vi "MainGUI.vi"() -> ()   [LabVIEW 2018]
uses:
  General/Controls/ScanType.ctl
  General/Controls/Vibratome Parameters.ctl
  General/Controls/Imaging Parameters.ctl
  General/Controls/Scan Direction.ctl
  General/type defines/Alazar parameters.ctl
  Hardware Mfg/AlazarTech SDK/Controls/General Trigger Settings.ctl
  Hardware Mfg/AlazarTech SDK/Controls/Trigger Engine Controls.ctl
  Hardware Mfg/AlazarTech SDK/Controls/Alazar Device ID.ctl
  Hardware Mfg/AlazarTech SDK/Controls/Channel Input Controls.ctl
  Hardware Mfg/AlazarTech SDK/Controls/Alazar Acquisition Settings.ctl
  Hardware Mfg/AlazarTech SDK/Controls/Clock Controls.ctl
  General/Controls/Optical Parameters.ctl
  General/Controls/Translation Stage Parameters.ctl
  Hardware Mfg/Thorlabs Translation Stages/Controls/Translation Stage Cluster.ctl
  General/Controls/Translation Stage Types.ctl
  General/type defines/Manual Controls.ctl
  General/type defines/FFT parameters.ctl
  General/type defines/FFT mode.ctl
  General/type defines/Vibratome Param.ctl
  General/Controls/Queue Manager Actions.ctl
  General/Controls/MessagePacket.ctl
  General/Controls/QueueNames.ctl
  General/Controls/FGV Actions.ctl
  General/Controls/Save Bline to Mem Control.ctl
  General/Tile naming actions.ctl
  Hardware Mfg/Main Scan Processor Status.vi
  Hardware Mfg/Axsun Laser/Axsun action.ctl
panel:
  in  "Status":string
  in  "Quit":bool
  in  "Acquire":bool
  in  "Control Panel":T1(tab)
  in  "Optical Parameters":T2={"Obj. Focal Length [mm]"=45.0, "Scan Lens EFL[mm]"=59.5, "Tube Lens EFL[mm]"=205.0, "Galvo V Range (+/-)"=10.0, "Galvo Max Half Angle [Deg]"=19.0, "Max Galvo Range[%]"=0.0}
  in  "Galvo HW Parameters":T3={"Analog Out Channel"="GalvoCtrl/ao0,GalvoCtrl/ao1", "Min Voltage"=-10.0, "Max Voltage"=10.0, "Pixel Clock Source"="/GalvoCtrl/PFI0", "Sample Rate"=1000.0, "Line Clock Out Ch"="GalvoCtrl/port0/line0"}
  in  "Imaging Parameter":T4={"Raster Scan Direction"=enum."Uni Directional", "Pixel Dwell Time [Clock Cycles]"=1, "Flyback Time [Clock Cycles]"=150, "XY Center [um]"={"X"=550.0, "Y"=450.0}, "Pixel Step Size [um] X"=3.0, "XY Image Size"=enum."2048 x 2048", "Custom"=TRUE, "Custom Size"={"X"=1050, "Y"=30}, "Line Averages"=1, "Pixel Step Size [um] Y"=0.0} {"Pixel Step Size [um] Y" min=0.0 max=10.0 step=0.01; "Line Averages" min=1 max=30 step=1; "Flyback Time [Clock Cycles]" max=1000 step=1; "Pixel Step Size [um] X" min=0.0 max=100.0 step=0.01; "Custom Size"."Y" min=2 max=10000 step=1; "Custom Size"."X" min=1 max=30 step=1; "XY Center [um]"."Y" min=1.0 max=30.0 step=1.0; "XY Center [um]"."X" min=1.0 max=30.0 step=1.0; "Pixel Dwell Time [Clock Cycles]" max=10 step=1}
  in  "Scan Type":T6
  in  "Alazar parameters":T7={"Trigger Settings"={"General Trigger Settings"={"Trigger Operation"=0, "Coupling ID"=2, "Range ID"=2, "Delay"=0, "Timeout Ticks"=0, "Mode"=1, "Parameter"=1}, "Trigger Engine 1"={"Trigger Engine"=0, "Source"=2, "Slope"=1, "Level"=140}, "Trigger Engine 2"={"Trigger Engine"=1, "Source"=2, "Slope"=1, "Level"=2048}}, "Device ID"={"System ID"=1, "Board ID"=1}, "Ch A Input Control"={"Channel"=1, "Coupling"=2, "Range"=7, "Impedance"=2}, "Ch B Input Control"={"Channel"=2, "Coupling"=2, "Range"=7, "Impedance"=2}, "Acq Settings"={"Record Length"=1440, "Offset"=0, "Records Per Buffer"=1100, "Records Count (Records/Acq)"=2147483647, "Window Type"=1, "Footer"=0, "Samples per record"=2048, "Output Format"=11}, "Capture Clock"={"Sample Rate"=100, "Decimation"=0, "Source"=2, "Edge"=0}} {"Capture Clock"."Edge" items=["Rising", "Falling"]; "Capture Clock"."Source" items=["Internal"=1, "Fast External"=2, "Medium External"=3, "Slow External"=4, "External AC"=5, "External DC"=6, "External 10MHz"=7]; "Acq Settings"."Output Format" items=["Float Log"=11, "Float Amp"=10, "U16_LOG"=1, "U16_AMP2"=257, "Real"=3, "Imag"=4]; "Acq Settings"."Footer" items=["FOOTER_NONE", "FOOTER_NPT"]; "Acq Settings"."Window Type" items=["DSP_WINDOW_NONE", "DSP_WINDOW_HANNING", "DSP_WINDOW_HAMMING", "DSP_WINDOW_BLACKMAN", "DSP_WINDOW_BLACKMAN_HARRIS", "DSP_WINDOW_BARTLETT"]; "Ch B Input Control"."Channel" items=["A"=1, "B"=2, "C"=4, "D"=8]; "Ch B Input Control"."Coupling" items=["AC"=1, "DC"=2]; "Ch B Input Control"."Range" items=["20 mV"=1, "40 mV"=2, "50 mV"=3, "80 mV"=4, "100 mV"=5, "200 mV"=6, "400 mV"=7, "500 mV"=8, "800 mV"=9, "1 V"=10, "1.25 V"=33, "2 V"=11, "4 V"=12, "5 V"=13, "8 V"=14, "10 V"=15, "20 V"=16]; "Ch B Input Control"."Impedance" items=["1 MOhm"=1, "50 Ohm"=2, ""=0]; "Ch A Input Control"."Channel" items=["A"=1, "B"=2, "C"=4, "D"=8]; "Ch A Input Control"."Coupling" items=["AC"=1, "DC"=2]; "Ch A Input Control"."Range" items=["20 mV"=1, "40 mV"=2, "50 mV"=3, "80 mV"=4, "100 mV"=5, "200 mV"=6, "400 mV"=7, "500 mV"=8, "800 mV"=9, "1 V"=10, "1.25 V"=33, "2 V"=11, "4 V"=12, "5 V"=13, "8 V"=14, "10 V"=15, "20 V"=16]; "Ch A Input Control"."Impedance" items=["1 MOhm"=1, "50 Ohm"=2, ""=0]; "Trigger Settings"."General Trigger Settings"."Trigger Operation" items=["J", "K", "J OR K", "J AND K", "J XOR K", "J AND NOT K", "NOT J AND K"]; "Trigger Settings"."General Trigger Settings"."Coupling ID" items=["AC"=1, "DC"=2]; "Trigger Settings"."General Trigger Settings"."Range ID" items=["5 V", "1 V", "TTL"]; "Trigger Settings"."Trigger Engine 1"."Trigger Engine" items=["J", "K"]; "Trigger Settings"."Trigger Engine 1"."Source" items=["A", "B", "External", "Disable", "C", "D"]; "Trigger Settings"."Trigger Engine 1"."Slope" items=["Positive"=1, "Negative"=2]; "Trigger Settings"."Trigger Engine 2"."Trigger Engine" items=["J", "K"]; "Trigger Settings"."Trigger Engine 2"."Source" items=["A", "B", "External", "Disable", "C", "D"]; "Trigger Settings"."Trigger Engine 2"."Slope" items=["Positive"=1, "Negative"=2]}
  in  "Vibratome Axis":T14={"Start [mm](first cut height)"=45.85, "slice thickness[um]"=2.1, "#slice"=111, "slice thick2[um]"=2.1, "#thin slices"=111, "image thickness(um)"=0.0, "#images"=0, "image depth2"=0.0, "#image depth2"=0}
  in  "Vibratome":T15={"Z Bottom [mm]"=0.0, "Pre Cut Dwell [s]"=0.0, "Blade Frequency [RPM]"=0, "Slice Speed [mm/s]"=0.0, "Post Cut Dwell [s]"=0.0, "Ramp Time [s]"=0.0, "Start X [mm]"=0.0, "Start Y [mm]"=0.0, "Slice Length [mm]"=0.0, "Slice Axis"=enum."X Axis", "Controller VISA Ref"="COM4"}
  in  "Mosaic Paramter":T16={"X Axis"={"Start [mm]"=56.0, "FOV[mm]"=3.0, "End [mm]"=70.8}, "Y Axis"={"Start [mm]"=102.5, "FOV[mm]"=3.0, "End [mm]"=117.2}, "Scan Pattern"=enum."Uni-directional", "Overlap Options"={"Overlap Type"=enum."X and Y", "Percent Overlap"=10, "Justify"=enum."Start"}}
  out "Current Position out":cluster{"X":dbl, "Y":dbl}
  in  "Manual Controls":T17={"Z0"=10.0, "First image height"=0.0, "Data Path"=path "C:/Users/BOAS-USER/Documents/Data/0922", "Save parameters"={"start pixel"=45, "#pixels to save"=100}, "Center Galvos"=FALSE, "Acquisition mode"=enum."Alazar FFT", "PSOCT Channel"=1, "Save"=FALSE, "AIP rotation angle"=0.0, "Scan Parameters"={"# Scan"={"#Ascan"=150, "#Bscan"=400}, "# Rpt"={"#ARpt"=1, "#BRpt"=1}, "Aline Rate"=2, "# Extra"={"# ARpt_extra"=5, "#Brtn_extra"=60}}, "ROI Parameters"={"ROI (mm)"={"X (mm)"=1.0, "Y (mm)"=1.0}, "Shift (mm)"={"Xshift (mm)"=0.0, "Yshift (mm)"=0.0}}, "Objective"=30} {"Objective" items=["5X LKM05", "10X LKM10", "20X LKM20", "10X LSM02"]; "Scan Parameters"."Aline Rate" items=["76 KHz", "146 KHz", "76 KHz", "28 KHz", "10 KHz"]; "PSOCT Channel" items=["A"=1, "B"=2, "A + B"=3, "C"=4, "A + C"=5, "A + B"=6, "D"=8, "A + D"=9, "B + D"=10, "C + D"=12, "A + B + C + D"=15]}
  out "image plane out":dbl
  out "slice plane out":dbl
  in  "Table Stages":T20={"X Stage"={"Position"=0.0, "Is.Enabled?"=FALSE, "Is.Connected?"=FALSE, "Device SN"="45876425", "AccelerationMaximum"=20.0, "VelocityMaximum"=20.0, "Acceleration"=10.0, "Velocity"=10.0, "waitTimeout (ms)"=1000000, "Model"=enum."Thorlabs LTS", "Is.Homed?"=FALSE}, "Y Stage"={"Position"=0.0, "Is.Enabled?"=FALSE, "Is.Connected?"=FALSE, "Device SN"="45995820", "AccelerationMaximum"=20.0, "VelocityMaximum"=20.0, "Acceleration"=10.0, "Velocity"=10.0, "waitTimeout (ms)"=10000000, "Model"=enum."Thorlabs LTS", "Is.Homed?"=FALSE}, "Z Stage"={"Position"=0.0, "Is.Enabled?"=FALSE, "Is.Connected?"=FALSE, "Device SN"="49103464", "AccelerationMaximum"=8.0, "VelocityMaximum"=3.0, "Acceleration"=4.0, "Velocity"=2.0, "waitTimeout (ms)"=1000000, "Model"=enum."Thorlabs MLJ", "Is.Homed?"=FALSE}}
  out "XY Graph out":cluster{"X":dbl, "Y":dbl}[](graph)
  out "AIP":T23(plugin-control) caption="Image"
  # "Image Settings"
  # "Optical Settings"
  # "X"
  # "X"
  # "Vibratome Settings"
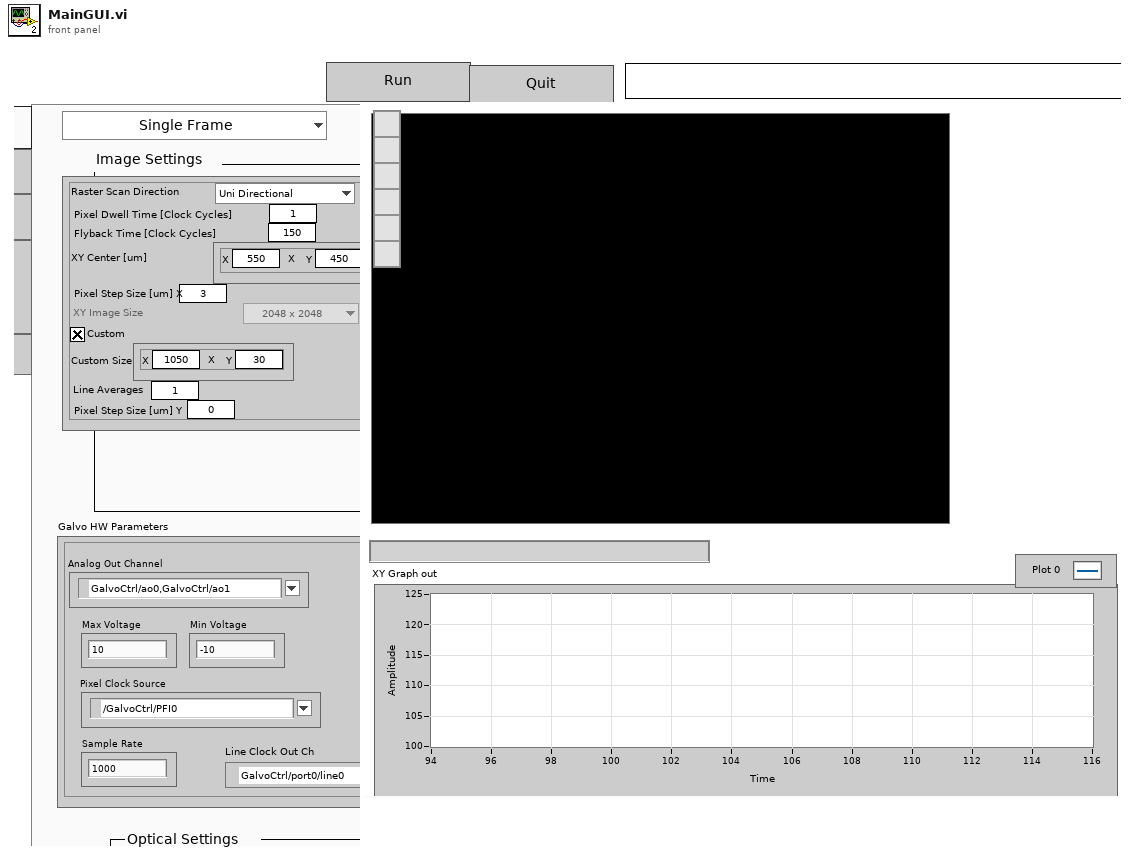
[diagram p1: front panel]
types:
  T1 = enum32{"Galvo", "Alazar", "Config", "Manual Contorls", "Table"}
  T2 = typedef "Optical Parameters.ctl" = cluster{"Obj. Focal Length [mm]":dbl, "Scan Lens EFL[mm]":dbl, "Tube Lens EFL[mm]":dbl, "Galvo V Range (+/-)":dbl, "Galvo Max Half Angle [Deg]":dbl, "Max Galvo Range[%]":dbl}
  T3 = cluster{"Analog Out Channel":tag, "Min Voltage":dbl, "Max Voltage":dbl, "Pixel Clock Source":tag, "Sample Rate":dbl, "Line Clock Out Ch":tag}
  T4 = typedef "Imaging Parameters.ctl" = cluster{"Raster Scan Direction":T5, "Pixel Dwell Time [Clock Cycles]":u16, "Flyback Time [Clock Cycles]":u16, "XY Center [um]":cluster{"X":dbl, "Y":dbl}, "Pixel Step Size [um] X":dbl, "XY Image Size":enum16{"32 x 32", "64 x 64", "128 x 128", "256 x 256", "512 x 512", "1024 x 1024", "2048 x 2048"}, "Custom":bool, "Custom Size":cluster{"X":u16, "Y":u16}, "Line Averages":u8, "Pixel Step Size [um] Y":dbl}
  T5 = typedef "Scan Direction.ctl" = enum16{"Uni Directional", "Bi Directional", "None"}
  T6 = typedef "ScanType.ctl" = enum16{"Single Frame", "Continuous Frame", "ROI Line", "Vibratome", "Mosaic", "Mosaic + Slice"}
  T7 = typedef "Alazar parameters.ctl" = cluster{"Trigger Settings":cluster{"General Trigger Settings":T8, "Trigger Engine 1":T9, "Trigger Engine 2":T9}, "Device ID":T10, "Ch A Input Control":T11, "Ch B Input Control":T11, "Acq Settings":T12, "Capture Clock":T13}
  T8 = typedef "General Trigger Settings.ctl" = cluster{"Trigger Operation":u32, "Coupling ID":u32, "Range ID":u32, "Delay":u32, "Timeout Ticks":u32, "Mode":u32, "Parameter":u32}
  T9 = typedef "Trigger Engine Controls.ctl" = cluster{"Trigger Engine":u32, "Source":u32, "Slope":u32, "Level":u32}
  T10 = typedef "Alazar Device ID.ctl" = cluster{"System ID":u32, "Board ID":u32}
  T11 = typedef "Channel Input Controls.ctl" = cluster{"Channel":u8, "Coupling":u32, "Range":u32, "Impedance":u32}
  T12 = typedef "Alazar Acquisition Settings.ctl" = cluster{"Record Length":u32, "Offset":u32, "Records Per Buffer":u32, "Records Count (Records/Acq)":u32, "Window Type":u32, "Footer":u32, "Samples per record":u32, "Output Format":u32}
  T13 = typedef "Clock Controls.ctl" = cluster{"Sample Rate":u32, "Decimation":u32, "Source":u32, "Edge":u32}
  T14 = typedef "Vibratome Param.ctl" = cluster{"Start [mm](first cut height)":dbl, "slice thickness[um]":dbl, "#slice":u16, "slice thick2[um]":dbl, "#thin slices":u16, "image thickness(um)":dbl, "#images":u16, "image depth2":dbl, "#image depth2":u16}
  T15 = typedef "Vibratome Parameters.ctl" = cluster{"Z Bottom [mm]":dbl, "Pre Cut Dwell [s]":dbl, "Blade Frequency [RPM]":u16, "Slice Speed [mm/s]":dbl, "Post Cut Dwell [s]":dbl, "Ramp Time [s]":dbl, "Start X [mm]":dbl, "Start Y [mm]":dbl, "Slice Length [mm]":dbl, "Slice Axis":enum16{"X Axis", "Y Axis", "Z Axis"}, "Controller VISA Ref":refnum<visa-resource-name>}
  T16 = cluster{"X Axis":cluster{"Start [mm]":dbl, "FOV[mm]":dbl, "End [mm]":dbl}, "Y Axis":cluster{"Start [mm]":dbl, "FOV[mm]":dbl, "End [mm]":dbl}, "Scan Pattern":enum16{"Uni-directional", "Bi-Directional", "Spiral Out", "Spiral In"}, "Overlap Options":cluster{"Overlap Type":enum16{"No Overlap", "X Only", "Y Only", "X and Y"}, "Percent Overlap":u8, "Justify":enum16{"Start", "Center", "End"}}}
  T17 = typedef "Manual Controls.ctl" = cluster{"Z0":dbl, "First image height":dbl, "Data Path":path, "Save parameters":T18, "Center Galvos":bool, "Acquisition mode":T19, "PSOCT Channel":u32, "Save":bool, "AIP rotation angle":dbl, "Scan Parameters":cluster{"# Scan":cluster{"#Ascan":i32, "#Bscan":i32}, "# Rpt":cluster{"#ARpt":i32, "#BRpt":i32}, "Aline Rate":u16, "# Extra":cluster{"# ARpt_extra":i32, "#Brtn_extra":i32}}, "ROI Parameters":cluster{"ROI (mm)":cluster{"X (mm)":dbl, "Y (mm)":dbl}, "Shift (mm)":cluster{"Xshift (mm)":sgl, "Yshift (mm)":sgl}}, "Objective":u16}
  T18 = typedef "FFT parameters.ctl" = cluster{"start pixel":i32, "#pixels to save":i32}
  T19 = typedef "FFT mode.ctl" = enum16{"ThorOCT B line", "ThorOCT Spectral", "ThorOCT FFT", "Alazar B line", "Alazar FFT", "GPU FFT", "Alazar Spectral"}
  T20 = typedef "Translation Stage Parameters.ctl" = cluster{"X Stage":T21, "Y Stage":T21, "Z Stage":T21}
  T21 = typedef "Translation Stage Cluster.ctl" = cluster{"Position":dbl, "Is.Enabled?":bool, "Is.Connected?":bool, "Device SN":string, "AccelerationMaximum":dbl, "VelocityMaximum":dbl, "Acceleration":dbl, "Velocity":dbl, "waitTimeout (ms)":i32, "Model":T22, "Is.Homed?":bool}
  T22 = typedef "Translation Stage Types.ctl" = enum16{"None", "Thorlabs LTS", "Thorlabs MLJ"}
  T23 = typedef "IMAQ Image.ctl" = refnum<image>
  T24 = typedef "Queue Manager Actions.ctl" = enum16{"Init", "Enqueue", "Enqueue All", "Preview Queue", "Dequeue", "Get Status", "Flush Queue", "Flush All Queues", "Release All Queues", "Release Queue", "Enqueue at Opposite End"}
  T25 = typedef "QueueNames.ctl" = enum16{"Main GUI", "Main Scan Processor", "Main Processing", "Main Saving", "Main Display", "Main Table Stage GUI", "Main Table Stage Proc.", "Scan Engine", "Vibratome GUI", "Vibratome Processor", "Slice Engine"}
  T26 = typedef "MessagePacket.ctl" = cluster{"Message":string, "Parameter":variant}
  T27 = typedef "FGV Actions.ctl" = enum16{"Init", "Set", "Get", "Clear"}
  T28 = typedef "Image Type" = u32
  T29 = typedef "System Parameters.ctl" = cluster{"Optical Parameters":T2, "Vibratome":T15, "Table Stages":T20, "Imaging Parameter":T4, "Galvo HW Parameters":cluster{"Analog Out Channel":tag, "Min Voltage":dbl, "Max Voltage":dbl, "Pixel Clock Source":tag, "Sample Rate":dbl, "Line Clock Out Ch":tag}, "Alazar parameters":T7, "Mosaic Paramter":cluster{"X Axis":cluster{"Start [mm]":dbl, "Steps [pts]":dbl, "End [mm]":dbl}, "Y Axis":cluster{"Start [mm]":dbl, "Steps [pts]":dbl, "End [mm]":dbl}, "Scan Pattern":enum16{"Uni-directional", "Bi-Directional", "Spiral Out", "Spiral In"}, "Overlap Options":cluster{"Overlap Type":enum16{"No Overlap", "X Only", "Y Only", "X and Y"}, "Percent Overlap":u8, "Justify":enum16{"Start", "Center", "End"}}}, "Manual Controls":T17, "Vibratome Axis":T14}
  T30 = typedef "Tile naming actions.ctl" = enum16{"Export", "Increment", "Total tile num", "Init"}
  T31 = typedef "Axsun action.ctl" = enum16{"GetSystemStatus", "Clock delay", "GetLaserOnTime", "GetWaveLengthAtSweptTrigger", "Source current ON", "GetSerialNum", "GetControlVersion", "Laser ON", "Laser OFF", "Source current OFF", "Get laser handle", "Start Network Control Interface", "stop", "Create handle"}
  T32 = typedef "Save Bline to Mem Control.ctl" = enum16{"Output data", "Save(ThorOCT)", "Save(PSOCT)", "FFT and Save", "Uninit", "PSOCT Spectral buffer Set", "PSOCT Spatial buffer Set", "PSOCT Spectral buffer Init", "PSOCT Spatial buffer Init", "ThorOCT Spectral buffer Init", "ThorOCT Spatial buffer Init", "ThorOCT Spectral buffer Set", "ThorOCT Spatial buffer Set", "ThorOCT Spectral Save", "Alazar Spectral Save"}
  T33 = cluster{"X Axis":cluster{"Start [mm]":dbl, "Steps [pts]":dbl, "End [mm]":dbl}, "Y Axis":cluster{"Start [mm]":dbl, "Steps [pts]":dbl, "End [mm]":dbl}, "Scan Pattern":enum16{"Uni-directional", "Bi-Directional", "Spiral Out", "Spiral In"}, "Overlap Options":cluster{"Overlap Type":enum16{"No Overlap", "X Only", "Y Only", "X and Y"}, "Percent Overlap":u8, "Justify":enum16{"Start", "Center", "End"}}}
  T34 = enum16{"32 x 32", "64 x 64", "128 x 128", "256 x 256", "512 x 512", "1024 x 1024", "2048 x 2048"}
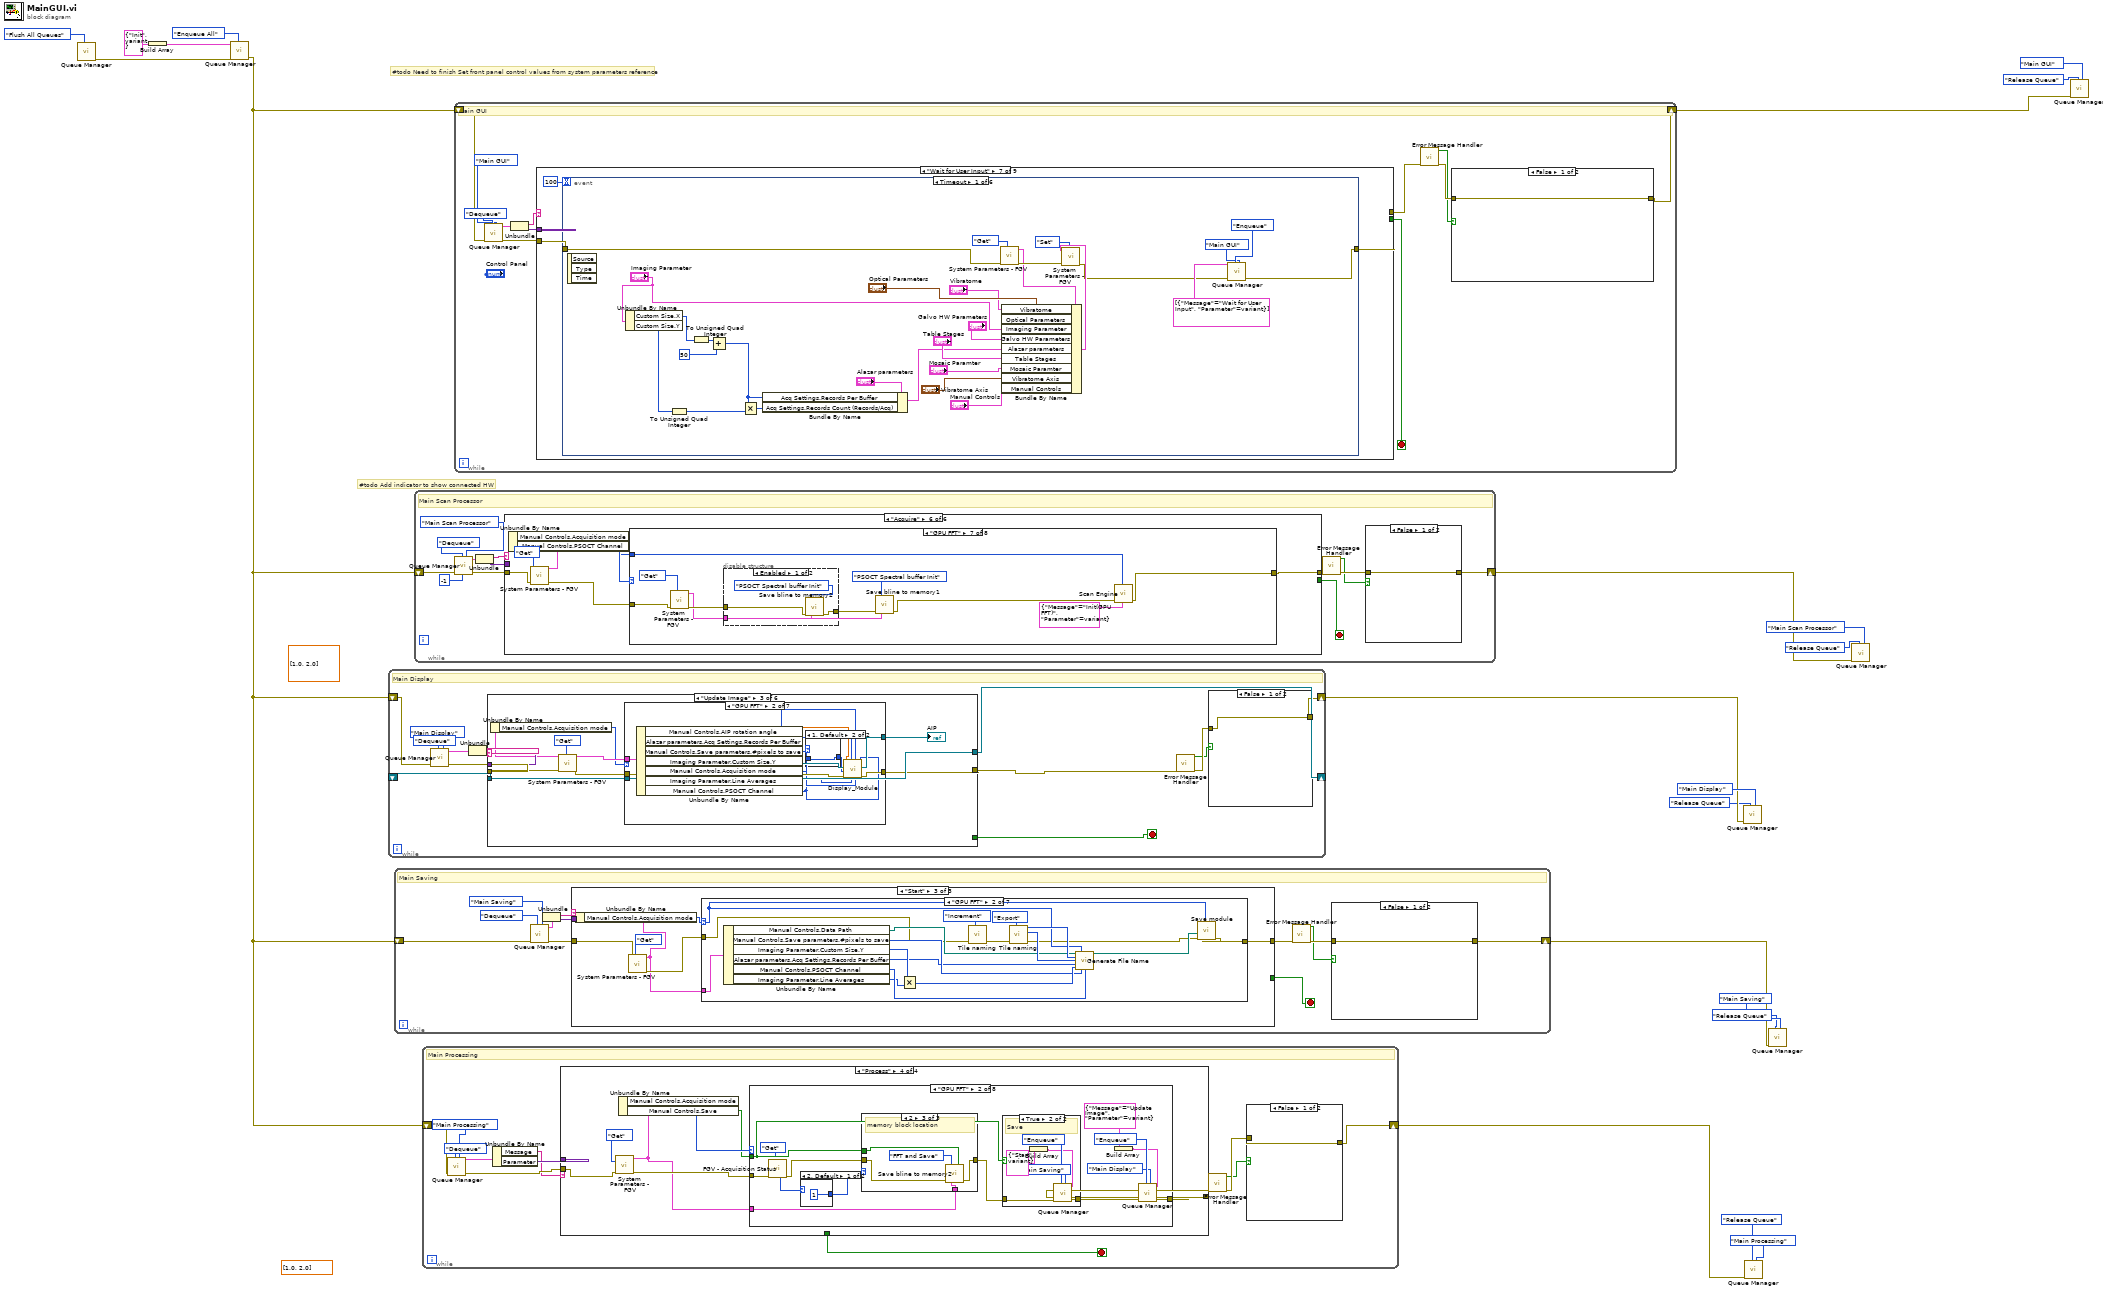
[diagram p0: block diagram]
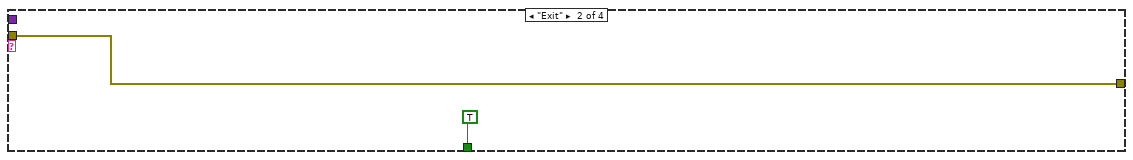
[diagram p3: hidden frame]
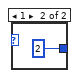
[diagram p6: hidden frame]
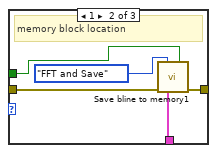
[diagram p9: hidden frame]
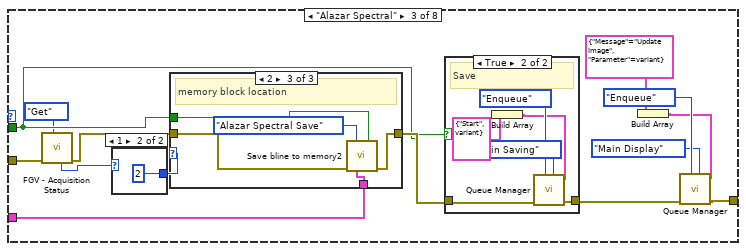
[diagram p10: hidden frame]
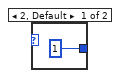
[diagram p11: hidden frame]
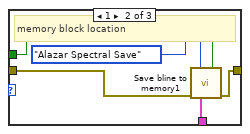
[diagram p14: hidden frame]
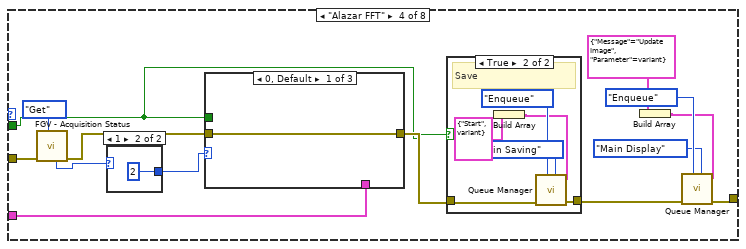
[diagram p15: hidden frame]
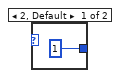
[diagram p16: hidden frame]
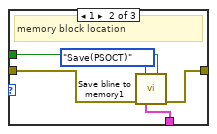
[diagram p18: hidden frame]
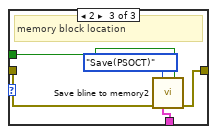
[diagram p19: hidden frame]
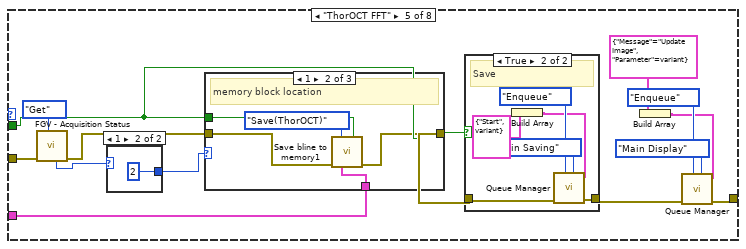
[diagram p20: hidden frame]
diagram:
  (unwired) dbl[] [1.0, 2.0]
  (unwired) dbl[][] [[1.0, 2.0]]
  # "#todo Add indicator to show connected HW"
  # "#todo Need to finish Set front panel control values from system parameters reference"
  n1 = call "Queue Manager.vi"("Action"=Queue_Manager_Actions."Flush All Queues") -> ("Error Out"=w1:errorcluster)  [unwired: 6 in, 4 out]
  n2 = Build Array(T26 {"Message"="Init", "Parameter"=variant} ("Message Packet [In]")) -> (w19:T26[])
  n3 = call "Queue Manager.vi"("Action"=Queue_Manager_Actions."Enqueue All", "Error In"=w1, "Message Packet Array"=w19) -> ("Error Out"=w4:errorcluster)  [unwired: 4 in, 4 out]
  n4 = while {
    shift-right: [w24] -> w11
    shift-left: w4 -> [w32]
    shift-right: [w34] -> _
    shift-left: _ -> [w33]
    stop <- w35 stop-if-true
    # "Main Display"
    n5 = call "Queue Manager.vi"("Queue Name"=QueueNames."Main Display", "Action"=Queue_Manager_Actions."Dequeue", "Error In"=w32) -> ("Error Out"=w29:errorcluster, "Message Packet [Out]"=w28:T26)  [unwired: 4 in, 3 out]
    n6 = Unbundle(w28) -> ("Message"=w27:string, "Parameter"=w26:variant)
    n7 = case shown="\"Update Image\"" w27 {
      tunnel: w29 -> [w46 w49 w67 w152 w154 w156]
      tunnel: w26 -> [_ _ _ _ _ _]
      tunnel: [w44 w50 w70 w144 w154 w156] -> w22
      tunnel: [TRUE _ _ _ _ _] -> w35
      tunnel: [_ w53 w72 w149 w153 w155] -> w34
      tunnel: w33 -> [_ _ w72 w149 w153 w155]
      frame "Exit" {
        n8 = call "RAW Image Buffer.vi"("Actions"=enum16{"Init", "Create", "Get", "Dispose"}."Dispose", "Error In"=w46) -> ("Error Out"=w45:errorcluster, "Image Out"=w42:T23)  [unwired: 8 in]
        n9 = local write "AIP"(w42) -> ()
        n10 = call "Image Queue.vi"("Action"=Queue_Manager_Actions."Release Queue", "Error In"=w45) -> ("Error Out"=w44:errorcluster)  [unwired: 8 in, 1 out]
      }
      frame "Init" {
        w54 = T28 2 items=["Grayscale (U8)", "Grayscale (I16)", "Grayscale (SGL)", "Complex (CSG)", "RGB (U32)", "HSL (U32)", "RGB (U64)", "Grayscale (U16)"] ("Image Type")
        n11 = call "RAW Image Buffer.vi"("Actions"=enum16{"Init", "Create", "Get", "Dispose"}."Init", "Error In"=w49) -> ("Error Out"=w58:errorcluster)  [unwired: 8 in, 1 out]
        n12 = call "RAW Image Buffer.vi"("Actions"=enum16{"Init", "Create", "Get", "Dispose"}."Create", "Error In"=w58) -> ("Error Out"=w52:errorcluster)  [unwired: 8 in, 1 out]
        n13 = disable-structure shown="Disabled" {
          disable-tunnel: w52 -> [w60 w64]
          disable-tunnel: [w59 w64] -> w51
          frame Disabled {
            n14 = call "Queue Manager.vi"("Queue Name"=QueueNames."Main Display", "Action"=Queue_Manager_Actions."Enqueue", "Error In"=w60, "Message Packet Array"=T26[] [{"Message"="Update Image", "Parameter"=variant}]) -> ("Error Out"=w59:errorcluster)  [unwired: 3 in, 4 out]
          }
          frame Enabled {
          }
        }
        n15 = call "IMAQ Create"("Image Name"="test", "Image Type"=w54, "error in (no error)"=w51) -> ("New Image"=w53:T23, "error out"=w50:errorcluster)  [unwired: 2 in]
      }
      frame "Update Image" {
        n16 = call "System Parameters - FGV.vi"("Actions"=FGV_Actions."Get", "Error In"=w67) -> ("Error Out"=w69:errorcluster, "System Parameters [Out]"=w66:T29)  [unwired: 8 in]
        n17 = Unbundle By Name(w66) -> ("Manual Controls.Acquisition mode"=w65:T19)
        n18 = case shown="\"GPU FFT\"" w65 {
          tunnel: w72 -> [w83 w96 w111 w124 w125 w139 w141]
          tunnel: [w82 w95 w110 w123 w125 w138 w141] -> w71
          tunnel: [w81 w94 w109 w122 w126 w137 w140] -> w70
          tunnel: w69 -> [w80 w93 w108 w121 w126 w136 w140]
          tunnel: w66 -> [w79 w92 w107 w120 _ w135 _]
          frame "Alazar FFT", Default {
            n19 = Unbundle By Name(w79) -> ("Manual Controls.AIP rotation angle"=w75:dbl, "Alazar parameters.Acq Settings.Records Per Buffer"=w76:u32, "Manual Controls.Save parameters.#pixels to save"=w78:i32, "Imaging Parameter.Custom Size.Y"=w77:u16, "Manual Controls.Acquisition mode"=w74:T19, "Imaging Parameter.Line Averages"=w73:u8)
            n20 = call "Display_Module.vi"("Acquisition mode"=w74, "Imaging Parameter.Line Averages"=w73, "Y"=w77, "X"=w76, "error in"=w80, "Z"=w78, "Source in"=w83, "Angle (degrees)"=w75) -> ("error out"=w81:errorcluster, "AIP"=w82:T23)  [unwired: 2 in]
          }
          frame "GPU FFT" {
            n21 = Unbundle By Name(w92) -> ("Manual Controls.AIP rotation angle"=w89:dbl, "Alazar parameters.Acq Settings.Records Per Buffer"=w90:u32, "Manual Controls.Save parameters.#pixels to save"=w85:i32, "Imaging Parameter.Custom Size.Y"=w91:u16, "Manual Controls.Acquisition mode"=w88:T19, "Imaging Parameter.Line Averages"=w87:u8, "Manual Controls.PSOCT Channel"=w86:u32)
            n22 = case shown="1, Default" w86 {
              tunnel: w85 -> [w99 w100]
              tunnel: [w98 w100] -> w84
              frame 3 {
                n23 = Multiply(x=2, y=w99) -> (x*y=w98:i32)
              }
              frame 1, Default {
              }
            }
            n24 = call "Display_Module.vi"("Manual Controls.PSOCT Channel"=w86, "Acquisition mode"=w88, "Imaging Parameter.Line Averages"=w87, "Y"=w91, "X"=w90, "error in"=w93, "Z"=w84, "Source in"=w96, "Angle (degrees)"=w89) -> ("error out"=w94:errorcluster, "AIP"=w95:T23)  [unwired: 1 in]
          }
          frame "Alazar B line" {
            n25 = Unbundle By Name(w107) -> ("Manual Controls.AIP rotation angle"=w103:dbl, "Alazar parameters.Acq Settings.Records Per Buffer"=w104:u32, "Manual Controls.Save parameters.#pixels to save"=w106:i32, "Imaging Parameter.Custom Size.Y"=w105:u16, "Manual Controls.Acquisition mode"=w102:T19, "Imaging Parameter.Line Averages"=w101:u8)
            n26 = call "Display_Module.vi"("Acquisition mode"=w102, "Imaging Parameter.Line Averages"=w101, "Y"=w105, "X"=w104, "error in"=w108, "Z"=w106, "Source in"=w111, "Angle (degrees)"=w103) -> ("error out"=w109:errorcluster, "AIP"=w110:T23)  [unwired: 2 in]
          }
          frame "ThorOCT FFT" {
            n27 = Unbundle By Name(w120) -> ("Manual Controls.AIP rotation angle"=w117:dbl, "Manual Controls.Scan Parameters.# Scan.#Ascan"=w113:i32, "Manual Controls.Save parameters.#pixels to save"=w119:i32, "Manual Controls.Scan Parameters.# Scan.#Bscan"=w118:i32, "Manual Controls.Acquisition mode"=w116:T19, "Manual Controls.Scan Parameters.# Extra.#Brtn_extra"=w114:i32)
            n28 = Add(x=w114, y=w113) -> (x+y=w112:i32)
            n29 = call "Display_Module.vi"("Acquisition mode"=w116, "Imaging Parameter.Line Averages"=1, "Y"=w118, "X"=w112, "error in"=w121, "Z"=w119, "Source in"=w124, "Angle (degrees)"=w117) -> ("error out"=w122:errorcluster, "AIP"=w123:T23)  [unwired: 2 in]
          }
          frame "ThorOCT Spectral" {
          }
          frame "ThorOCT B line" {
            n30 = Unbundle By Name(w135) -> ("Manual Controls.AIP rotation angle"=w132:dbl, "Manual Controls.Scan Parameters.# Scan.#Ascan"=w128:i32, "Manual Controls.Save parameters.#pixels to save"=w134:i32, "Manual Controls.Scan Parameters.# Scan.#Bscan"=w133:i32, "Manual Controls.Acquisition mode"=w131:T19, "Manual Controls.Scan Parameters.# Extra.#Brtn_extra"=w129:i32)
            n31 = Add(x=w129, y=w128) -> (x+y=w127:i32)
            n32 = call "Display_Module.vi"("Acquisition mode"=w131, "Imaging Parameter.Line Averages"=1, "Y"=w133, "X"=w127, "error in"=w136, "Z"=w134, "Source in"=w139, "Angle (degrees)"=w132) -> ("error out"=w137:errorcluster, "AIP"=w138:T23)  [unwired: 2 in]
          }
          frame "Alazar Spectral" {
          }
        }
        "AIP" <- w71
      }
      frame "Update Status" {
        n33 = call "Status Queue.vi"("Action"=Queue_Manager_Actions."Get Status", "Error In"=w152) -> ("Error Out"=w145:errorcluster, "Status Message [Out]"=w150:string)  [unwired: 8 in]
        n34 = local write "Status"(w150) -> ()
        n35 = call "Scan engine status.vi"("Actions"=FGV_Actions."Get", "Error In"=w145) -> ("slice plane out"=→"slice plane out":dbl, "image plane out"=→"image plane out":dbl, "XY Graph out"=→"XY Graph out":cluster{"X":dbl, "Y":dbl}[], "Current Position out"=→"Current Position out":cluster{"X":dbl, "Y":dbl}, "Error Out"=w144:errorcluster)  [unwired: 8 in, 1 out]
      }
      frame "Update Line Profile" {
      }
      frame "Idle", Default {
      }
    }
    n36 = call "Error Message Handler.vi"("Error In"=w22) -> ("Error Out"=w25:errorcluster, "T button?"=w23:bool)  [unwired: 9 in]
    n37 = case shown="False" w23 {
      tunnel: [w36 w39] -> w24
      tunnel: w25 -> [w36 w37]
      frame False {
      }
      frame True {
        n38 = call "Queue Manager.vi"("Queue Name"=QueueNames."Main Display", "Action"=Queue_Manager_Actions."Enqueue", "Error In"=w37, "Message Packet Array"=T26[] [{"Message"="Exit", "Parameter"=variant}] ("Message Packet [In]")) -> ("Error Out"=w39:errorcluster)  [unwired: 3 in, 4 out]
      }
    }
  }
  n39 = while {
    shift-right: [w160] -> w7
    shift-left: w4 -> [w157]
    stop <- w158 stop-if-true
    # "Main Saving"
    n40 = call "Queue Manager.vi"("Queue Name"=QueueNames."Main Saving", "Action"=Queue_Manager_Actions."Dequeue", "Error In"=w157) -> ("Error Out"=w164:errorcluster, "Message Packet [Out]"=w168:T26)  [unwired: 4 in, 3 out]
    n41 = Unbundle(w168) -> ("Message"=w159:string, "Parameter"=w165:variant)
    n42 = case shown="\"Start\"" w159 {
      tunnel: [w178 _ w185] -> w161
      tunnel: w165 -> [_ _ _]
      tunnel: w164 -> [w178 _ w183]
      tunnel: [_ TRUE _] -> w158
      frame "False", Default {
      }
      frame "Exit" {
      }
      frame "Start" {
        n43 = call "System Parameters - FGV.vi"("Actions"=FGV_Actions."Get", "Error In"=w183) -> ("Error Out"=w182:errorcluster, "System Parameters [Out]"=w181:T29)  [unwired: 8 in]
        n44 = Unbundle By Name(w181) -> ("Manual Controls.Acquisition mode"=w180:T19)
        n45 = case shown="\"GPU FFT\"" w180 {
          selector: w180 -> [w186 w206 w229 w245 w261 w277 w293]
          tunnel: [w201 w219 w226 w260 w276 w292 w308] -> w185
          tunnel: w182 -> [w195 w203 w232 w254 w270 w286 w302]
          tunnel: w181 -> [w193 w213 w231 w252 w269 w285 w301]
          frame "Alazar FFT", Default {
            n46 = Unbundle By Name(w193) -> ("Manual Controls.Data Path"=w191:path, "Manual Controls.Save parameters.#pixels to save"=w190:i32, "Imaging Parameter.Custom Size.Y"=w194:u16, "Alazar parameters.Acq Settings.Records Per Buffer"=w189:u32, "Manual Controls.PSOCT Channel"=w188:u32, "Imaging Parameter.Line Averages"=w187:u8)
            n47 = Multiply(x=w194, y=w187) -> (x*y=w192:u16)
            n48 = call "Tile naming.vi"(7:Tile_naming_actions."Export", "Error In"=w195) -> ("Error Out"=w196:errorcluster, "tile"=w197:i32, "slice"=w198:i32)  [unwired: 7 in]
            n49 = call "Generate File Name.vi"("stripped path"=w191, "Acquisition mode"=w186, "slice"=w198, "tile"=w197, "X"=w189, "Y"=w192, "Z"=w190, "Channel"=w188) -> ("appended path"=w200:path)  [unwired: 7 in]
            n50 = call "Save module.vi"("Acquisition mode"=w186, "error in"=w196, "path"=w200) -> ("error out"=w201:errorcluster)  [unwired: 8 in]
          }
          frame "GPU FFT" {
            n51 = Unbundle By Name(w213) -> ("Manual Controls.Data Path"=w211:path, "Manual Controls.Save parameters.#pixels to save"=w210:i32, "Imaging Parameter.Custom Size.Y"=w214:u16, "Alazar parameters.Acq Settings.Records Per Buffer"=w209:u32, "Manual Controls.PSOCT Channel"=w208:u32, "Imaging Parameter.Line Averages"=w207:u8)
            n52 = Multiply(x=w214, y=w207) -> (x*y=w212:u16)
            n53 = call "Tile naming.vi"(7:Tile_naming_actions."Increment", "Error In"=w203) -> ("Error Out"=w204:errorcluster)  [unwired: 7 in, 2 out]
            n54 = call "Tile naming.vi"(7:Tile_naming_actions."Export", "Error In"=w204) -> ("Error Out"=w202:errorcluster, "tile"=w215:i32, "slice"=w216:i32)  [unwired: 7 in]
            n55 = call "Generate File Name.vi"("stripped path"=w211, "Acquisition mode"=w206, "slice"=w216, "tile"=w215, "X"=w209, "Y"=w212, "Z"=w210, "Channel"=w208) -> ("appended path"=w218:path)  [unwired: 7 in]
            n56 = call "Save module.vi"("Acquisition mode"=w206, "error in"=w202, "path"=w218) -> ("error out"=w219:errorcluster)  [unwired: 8 in]
          }
          frame "Alazar Spectral" {
            n57 = Unbundle By Name(w231) -> ("Manual Controls.Data Path"=w230:path, "Imaging Parameter.Custom Size.Y"=w223:u16, "Alazar parameters.Acq Settings.Records Per Buffer"=w228:u32, "Manual Controls.PSOCT Channel"=w225:u32, "Imaging Parameter.Line Averages"=w222:u8)  [unwired: 1 out]
            n58 = case shown="3" w225 {
              tunnel: [1 2] -> w221
              frame 1, Default {
              }
              frame 3 {
              }
            }
            n59 = Compound Arithmetic op=MULTIPLY(w223, w222, w221) -> (w220:i32)
            n60 = call "Tile naming.vi"(7:Tile_naming_actions."Export", "Error In"=w232) -> ("Error Out"=w233:errorcluster, "tile"=w234:i32, "slice"=w235:i32)  [unwired: 7 in]
            n61 = call "Generate File Name.vi"("stripped path"=w230, "Acquisition mode"=w229, "slice"=w235, "tile"=w234, "X"=w228, "Y"=w220, "Z"=1440, "Channel"=w225) -> ("appended path"=w237:path)  [unwired: 7 in]
            n62 = call "Save module.vi"("Acquisition mode"=w229, "error in"=w233, "path"=w237, "#A lines"=w228, "#B lines"=w220) -> ("error out"=w227:errorcluster)  [unwired: 6 in]
            n63 = disable-structure shown="Enabled" {
              disable-tunnel: w227 -> [w241 w242]
              disable-tunnel: [w240 w242] -> w226
              frame Disabled {
                n64 = call "Process status.vi"("Actions"=FGV_Actions."Set", "Error In"=w241, "Status In"=TRUE) -> ("Error Out"=w240:errorcluster)  [unwired: 7 in, 1 out]
              }
              frame Enabled {
              }
            }
          }
          frame "Alazar B line" {
            n65 = Unbundle By Name(w252) -> ("Manual Controls.Data Path"=w250:path, "Manual Controls.Save parameters.#pixels to save"=w249:i32, "Imaging Parameter.Custom Size.Y"=w253:u16, "Alazar parameters.Acq Settings.Records Per Buffer"=w248:u32, "Manual Controls.PSOCT Channel"=w247:u32, "Imaging Parameter.Line Averages"=w246:u8)
            n66 = Multiply(x=w253, y=w246) -> (x*y=w251:u16)
            n67 = call "Tile naming.vi"(7:Tile_naming_actions."Export", "Error In"=w254) -> ("Error Out"=w255:errorcluster, "tile"=w256:i32, "slice"=w257:i32)  [unwired: 7 in]
            n68 = call "Generate File Name.vi"("stripped path"=w250, "Acquisition mode"=w245, "slice"=w257, "tile"=w256, "X"=w248, "Y"=w251, "Z"=w249, "Channel"=w247) -> ("appended path"=w259:path)  [unwired: 7 in]
            n69 = call "Save module.vi"("Acquisition mode"=w245, "error in"=w255, "path"=w259) -> ("error out"=w260:errorcluster)  [unwired: 8 in]
          }
          frame "ThorOCT FFT" {
            n70 = Unbundle By Name(w269) -> ("Manual Controls.Data Path"=w268:path, "Manual Controls.Save parameters.#pixels to save"=w267:i32, "Manual Controls.Scan Parameters.# Scan.#Bscan"=w262:i32, "Manual Controls.Scan Parameters.# Scan.#Ascan"=w265:i32, "Manual Controls.PSOCT Channel"=w266:u32, "Manual Controls.Scan Parameters.# Extra.#Brtn_extra"=w264:i32)
            n71 = Add(x=w265, y=w264) -> (x+y=w263:i32)
            n72 = call "Tile naming.vi"(7:Tile_naming_actions."Export", "Error In"=w270) -> ("Error Out"=w271:errorcluster, "tile"=w272:i32, "slice"=w273:i32)  [unwired: 7 in]
            n73 = call "Generate File Name.vi"("stripped path"=w268, "Acquisition mode"=w261, "slice"=w273, "tile"=w272, "X"=w263, "Y"=w262, "Z"=w267, "Channel"=w266) -> ("appended path"=w275:path)  [unwired: 7 in]
            n74 = call "Save module.vi"("Acquisition mode"=w261, "error in"=w271, "path"=w275) -> ("error out"=w276:errorcluster)  [unwired: 8 in]
          }
          frame "ThorOCT Spectral" {
            n75 = Unbundle By Name(w285) -> ("Manual Controls.Data Path"=w284:path, "Manual Controls.Scan Parameters.# Scan.#Bscan"=w279:i32, "Manual Controls.Scan Parameters.# Scan.#Ascan"=w282:i32, "Manual Controls.PSOCT Channel"=w283:u32, "Manual Controls.Scan Parameters.# Extra.#Brtn_extra"=w281:i32)  [unwired: 1 out]
            n76 = Add(x=w282, y=w281) -> (x+y=w280:i32)
            n77 = call "Tile naming.vi"(7:Tile_naming_actions."Export", "Error In"=w286) -> ("Error Out"=w287:errorcluster, "tile"=w288:i32, "slice"=w289:i32)  [unwired: 7 in]
            n78 = call "Generate File Name.vi"("stripped path"=w284, "Acquisition mode"=w277, "slice"=w289, "tile"=w288, "X"=w280, "Y"=w279, "Z"=2048, "Channel"=w283) -> ("appended path"=w291:path)  [unwired: 7 in]
            n79 = call "Save module.vi"("Acquisition mode"=w277, "error in"=w287, "path"=w291) -> ("error out"=w292:errorcluster)  [unwired: 8 in]
          }
          frame "ThorOCT B line" {
            n80 = Unbundle By Name(w301) -> ("Manual Controls.Data Path"=w300:path, "Manual Controls.Save parameters.#pixels to save"=w299:i32, "Manual Controls.Scan Parameters.# Scan.#Bscan"=w294:i32, "Manual Controls.Scan Parameters.# Scan.#Ascan"=w297:i32, "Manual Controls.PSOCT Channel"=w298:u32, "Manual Controls.Scan Parameters.# Extra.#Brtn_extra"=w296:i32)
            n81 = Add(x=w297, y=w296) -> (x+y=w295:i32)
            n82 = call "Tile naming.vi"(7:Tile_naming_actions."Export", "Error In"=w302) -> ("Error Out"=w303:errorcluster, "tile"=w304:i32, "slice"=w305:i32)  [unwired: 7 in]
            n83 = call "Generate File Name.vi"("stripped path"=w300, "Acquisition mode"=w293, "slice"=w305, "tile"=w304, "X"=w295, "Y"=w294, "Z"=w299, "Channel"=w298) -> ("appended path"=w307:path)  [unwired: 7 in]
            n84 = call "Save module.vi"("Acquisition mode"=w293, "error in"=w303, "path"=w307) -> ("error out"=w308:errorcluster)  [unwired: 8 in]
          }
        }
      }
    }
    n85 = call "Error Message Handler.vi"("Error In"=w161) -> ("Error Out"=w163:errorcluster, "T button?"=w162:bool)  [unwired: 9 in]
    n86 = case shown="False" w162 {
      tunnel: [w169 w175] -> w160
      tunnel: w163 -> [w169 w171]
      frame False {
      }
      frame True {
        n87 = call "Queue Manager.vi"("Queue Name"=QueueNames."Main Saving", "Action"=Queue_Manager_Actions."Flush Queue", "Error In"=w171) -> ("Error Out"=w170:errorcluster)  [unwired: 4 in, 4 out]
        n88 = call "Queue Manager.vi"("Queue Name"=QueueNames."Main Saving", "Action"=Queue_Manager_Actions."Enqueue", "Error In"=w170, "Message Packet Array"=T26[] [{"Message"="Exit", "Parameter"=variant}] ("Message Packet [In]")) -> ("Error Out"=w175:errorcluster)  [unwired: 3 in, 4 out]
      }
    }
  }
  n89 = while {
    shift-right: [w311] -> w13
    shift-left: w4 -> [w320]
    stop <- w321 stop-if-true
    # "Main Scan Processor"
    n90 = call "Queue Manager.vi"("Queue Name"=QueueNames."Main Scan Processor", "timeout in ms (-1)"=-1, "Action"=Queue_Manager_Actions."Dequeue", "Error In"=w320) -> ("Error Out"=w310:errorcluster, "Message Packet [Out]"=w318:T26)  [unwired: 3 in, 3 out]
    n91 = Unbundle(w318) -> ("Message"=w317:string, "Parameter"=w316:variant)
    n92 = case shown="\"Acquire\"" w317 {
      tunnel: w316 -> [_ _ _ _ _ _]
      tunnel: [w322 w324 w330 w332 w346 w354] -> w314
      tunnel: [TRUE _ _ _ _ _] -> w321
      tunnel: w310 -> [w322 w324 w326 w331 w346 w352]
      frame "Exit" {
      }
      frame "Init" {
      }
      frame "Init Hardware" {
        n93 = global write "Main Scan Processor Status.vi" "Busy"(TRUE ("Busy")) -> ()
        n94 = call "Queue Manager.vi"("Queue Name"=QueueNames."Main Scan Processor", "Action"=Queue_Manager_Actions."Enqueue", "Error In"=w326, "Message Packet Array"=T26[] [{"Message"="Init Laser", "Parameter"=variant}, {"Message"="", "Parameter"=variant}, {"Message"="", "Parameter"=variant}, {"Message"="", "Parameter"=variant}, {"Message"="", "Parameter"=variant}, {"Message"="", "Parameter"=variant}, {"Message"="", "Parameter"=variant}]) -> ("Error Out"=w330:errorcluster)  [unwired: 3 in, 4 out]
      }
      frame "Init Laser" {
        n95 = disable-structure shown="Disabled" {
          disable-tunnel: w331 -> [w334 _]
          disable-tunnel: [w333 _] -> w332
          frame Disabled {
            n96 = call "Axsun module.vi"("Action"=Axsun_action."Create handle", "error in (no error)"=w334) -> ("error out"=w344:errorcluster)  [unwired: 8 in, 1 out]
            n97 = call "Axsun module.vi"("Action"=Axsun_action."GetControlVersion", "error in (no error)"=w344) -> ("error out"=w343:errorcluster)  [unwired: 8 in, 1 out]
            n98 = call "Axsun module.vi"("Action"=Axsun_action."Start Network Control Interface", "error in (no error)"=w343) -> ("error out"=w342:errorcluster)  [unwired: 8 in, 1 out]
            n99 = call "Axsun module.vi"("Action"=Axsun_action."Get laser handle", "error in (no error)"=w342) -> ("error out"=w341:errorcluster)  [unwired: 8 in, 1 out]
            n100 = call "Axsun module.vi"("Action"=Axsun_action."GetSerialNum", "error in (no error)"=w341) -> ("error out"=w340:errorcluster)  [unwired: 8 in, 1 out]
            n101 = call "Axsun module.vi"("Action"=Axsun_action."GetSystemStatus", "error in (no error)"=w340) -> ("error out"=w333:errorcluster)  [unwired: 8 in, 1 out]
          }
          frame Enabled {
          }
        }
      }
      frame "Idle", Default {
        n102 = global write "Main Scan Processor Status.vi" "Busy"(FALSE ("Busy")) -> ()
      }
      frame "Acquire" {
        n103 = call "System Parameters - FGV.vi"("Actions"=FGV_Actions."Get", "Error In"=w352) -> ("Error Out"=w351:errorcluster, "System Parameters [Out]"=w350:T29)  [unwired: 8 in]
        n104 = Unbundle By Name(w350) -> ("Manual Controls.Acquisition mode"=w349:T19, "Manual Controls.PSOCT Channel"=w348:u32)
        n105 = case shown="\"GPU FFT\"" w349 {
          tunnel: [w355 w359 w369 w379 w397 w409 w417 w433] -> w354
          tunnel: w351 -> [w355 w362 w372 w382 w389 w402 w415 w431]
          tunnel: w348 -> [_ _ _ _ w392 w405 w412 w428]
          frame Default {
          }
          frame "ThorOCT Spectral" {
            n106 = call "System Parameters - FGV.vi"("Actions"=FGV_Actions."Get", "Error In"=w362) -> ("Error Out"=w363:errorcluster, "System Parameters [Out]"=w357:T29)  [unwired: 8 in]
            n107 = call "Save bline to memory2.vi"("action"=Save_Bline_to_Mem_Control."ThorOCT Spectral buffer Init", "error in"=w363, "System Parameters"=w357) -> ("error out"=w365:errorcluster)  [unwired: 12 in]
            n108 = call "Save bline to memory1.vi"("action"=Save_Bline_to_Mem_Control."ThorOCT Spectral buffer Init", "error in"=w365, "System Parameters"=w357) -> ("error out"=w360:errorcluster)  [unwired: 12 in]
            n109 = call "Scan Engine.vi"("Message Packet"=T26 {"Message"="Init ThorOCT Spectral", "Parameter"=variant}, "Error In"=w360) -> ("Error Out"=w359:errorcluster)  [unwired: 9 in]
          }
          frame "ThorOCT FFT" {
            n110 = call "System Parameters - FGV.vi"("Actions"=FGV_Actions."Get", "Error In"=w372) -> ("Error Out"=w373:errorcluster, "System Parameters [Out]"=w367:T29)  [unwired: 8 in]
            n111 = call "Save bline to memory2.vi"("action"=Save_Bline_to_Mem_Control."ThorOCT Spatial buffer Init", "error in"=w373, "System Parameters"=w367) -> ("error out"=w375:errorcluster)  [unwired: 12 in]
            n112 = call "Save bline to memory1.vi"("action"=Save_Bline_to_Mem_Control."ThorOCT Spatial buffer Init", "error in"=w375, "System Parameters"=w367) -> ("error out"=w370:errorcluster)  [unwired: 12 in]
            n113 = call "Scan Engine.vi"("Message Packet"=T26 {"Message"="Init ThorOCT Spatial", "Parameter"=variant}, "Error In"=w370) -> ("Error Out"=w369:errorcluster)  [unwired: 9 in]
          }
          frame "ThorOCT B line" {
            n114 = call "System Parameters - FGV.vi"("Actions"=FGV_Actions."Get", "Error In"=w382) -> ("Error Out"=w383:errorcluster, "System Parameters [Out]"=w377:T29)  [unwired: 8 in]
            n115 = call "Save bline to memory2.vi"("action"=Save_Bline_to_Mem_Control."ThorOCT Spatial buffer Init", "error in"=w383, "System Parameters"=w377) -> ("error out"=w385:errorcluster)  [unwired: 12 in]
            n116 = call "Save bline to memory1.vi"("action"=Save_Bline_to_Mem_Control."ThorOCT Spatial buffer Init", "error in"=w385, "System Parameters"=w377) -> ("error out"=w380:errorcluster)  [unwired: 12 in]
            n117 = call "Scan Engine.vi"("Message Packet"=T26 {"Message"="Init ThorOCT Spatial", "Parameter"=variant}, "Error In"=w380) -> ("Error Out"=w379:errorcluster)  [unwired: 9 in]
          }
          frame "Alazar FFT" {
            # "Acquisition mode"
            n118 = call "System Parameters - FGV.vi"("Actions"=FGV_Actions."Get", "Error In"=w389) -> ("Error Out"=w388:errorcluster, "System Parameters [Out]"=w387:T29)  [unwired: 8 in]
            n119 = global write "Main Scan Processor Status.vi" "Busy"(TRUE ("Busy")) -> ()
            n120 = call "Save bline to memory2.vi"("action"=Save_Bline_to_Mem_Control."PSOCT Spatial buffer Init", "error in"=w388, "System Parameters"=w387) -> ("error out"=w394:errorcluster)  [unwired: 12 in]
            n121 = call "Save bline to memory1.vi"("action"=Save_Bline_to_Mem_Control."PSOCT Spatial buffer Init", "error in"=w394, "System Parameters"=w387) -> ("error out"=w391:errorcluster)  [unwired: 12 in]
            n122 = call "Scan Engine.vi"("Message Packet"=T26 {"Message"="Init(Alazar FFT)", "Parameter"=variant}, "Channel"=w392, "Error In"=w391) -> ("Error Out"=w397:errorcluster)  [unwired: 8 in]
          }
          frame "Alazar B line" {
            # "Acquisition mode"
            n123 = call "System Parameters - FGV.vi"("Actions"=FGV_Actions."Get", "Error In"=w402) -> ("Error Out"=w401:errorcluster, "System Parameters [Out]"=w398:T29)  [unwired: 8 in]
            n124 = global write "Main Scan Processor Status.vi" "Busy"(TRUE ("Busy")) -> ()
            n125 = call "Save bline to memory2.vi"("action"=Save_Bline_to_Mem_Control."PSOCT Spatial buffer Init", "error in"=w401, "System Parameters"=w398) -> ("error out"=w406:errorcluster)  [unwired: 12 in]
            n126 = call "Save bline to memory1.vi"("action"=Save_Bline_to_Mem_Control."PSOCT Spatial buffer Init", "error in"=w406, "System Parameters"=w398) -> ("error out"=w404:errorcluster)  [unwired: 12 in]
            n127 = call "Scan Engine.vi"("Message Packet"=T26 {"Message"="Init(Alazar FFT)", "Parameter"=variant}, "Channel"=w405, "Error In"=w404) -> ("Error Out"=w409:errorcluster)  [unwired: 8 in]
          }
          frame "GPU FFT" {
            n128 = call "System Parameters - FGV.vi"("Actions"=FGV_Actions."Get", "Error In"=w415) -> ("Error Out"=w414:errorcluster, "System Parameters [Out]"=w410:T29)  [unwired: 8 in]
            n129 = disable-structure shown="Enabled" {
              disable-tunnel: [w423 w424] -> w418
              disable-tunnel: w414 -> [w422 w424]
              disable-tunnel: w410 -> [w420 _]
              frame Enabled {
                n130 = call "Save bline to memory2.vi"("action"=Save_Bline_to_Mem_Control."PSOCT Spectral buffer Init", "error in"=w422, "System Parameters"=w420) -> ("error out"=w423:errorcluster)  [unwired: 12 in]
              }
              frame Disabled {
              }
            }
            n131 = call "Save bline to memory1.vi"("action"=Save_Bline_to_Mem_Control."PSOCT Spectral buffer Init", "error in"=w418, "System Parameters"=w410) -> ("error out"=w413:errorcluster)  [unwired: 12 in]
            n132 = call "Scan Engine.vi"("Message Packet"=T26 {"Message"="Init(GPU FFT)", "Parameter"=variant}, "Channel"=w412, "Error In"=w413) -> ("Error Out"=w417:errorcluster)  [unwired: 8 in]
          }
          frame "Alazar Spectral" {
            n133 = call "System Parameters - FGV.vi"("Actions"=FGV_Actions."Get", "Error In"=w431) -> ("Error Out"=w430:errorcluster, "System Parameters [Out]"=w425:T29)  [unwired: 8 in]
            n134 = call "Save bline to memory2.vi"("action"=Save_Bline_to_Mem_Control."PSOCT Spectral buffer Init", "error in"=w430, "System Parameters"=w425) -> ("error out"=w434:errorcluster)  [unwired: 12 in]
            n135 = call "Save bline to memory1.vi"("action"=Save_Bline_to_Mem_Control."PSOCT Spectral buffer Init", "error in"=w434, "System Parameters"=w425) -> ("error out"=w429:errorcluster)  [unwired: 12 in]
            n136 = call "Scan Engine.vi"("Message Packet"=T26 {"Message"="Init(GPU FFT)", "Parameter"=variant}, "Channel"=w428, "Error In"=w429) -> ("Error Out"=w433:errorcluster)  [unwired: 8 in]
          }
        }
      }
    }
    n137 = call "Error Message Handler.vi"("Error In"=w314) -> ("Error Out"=w313:errorcluster, "T button?"=w312:bool)  [unwired: 9 in]
    n138 = case shown="False" w312 {
      tunnel: w313 -> [w436 w438]
      tunnel: [w436 w439] -> w311
      frame False {
      }
      frame True {
        n139 = call "Queue Manager.vi"("Queue Name"=QueueNames."Main Scan Processor", "Action"=Queue_Manager_Actions."Enqueue", "Error In"=w438, "Message Packet Array"=T26[] [{"Message"="Exit", "Parameter"=variant}] ("Message Packet [In]")) -> ("Error Out"=w439:errorcluster)  [unwired: 3 in, 4 out]
      }
    }
  }
  n140 = while "Main Data Processing" {
    shift-right: [w449] -> w5
    shift-left: w4 -> [w453]
    stop <- w445 stop-if-true
    # "Main Processing"
    n141 = call "Queue Manager.vi"("Queue Name"=QueueNames."Main Processing", "Action"=Queue_Manager_Actions."Dequeue", "Error In"=w453) -> ("Error Out"=w444:errorcluster, "Message Packet [Out]"=w447:T26)  [unwired: 4 in, 3 out]
    n142 = Unbundle By Name(w447) -> ("Message"=w442:string, "Parameter"=w443:variant)
    n143 = case shown="\"Process\"" w442 {
      tunnel: [w454 w455 w457 w464] -> w446
      tunnel: [_ TRUE ("Exit") _ _] -> w445
      tunnel: w444 -> [w454 w455 w457 w462]
      tunnel: w443 -> [_ _ _ _]
      frame "False", Default {
      }
      frame "Exit" {
      }
      frame "Init" {
      }
      frame "Process" {
        n144 = call "System Parameters - FGV.vi"("Actions"=FGV_Actions."Get", "Error In"=w462) -> ("Error Out"=w461:errorcluster, "System Parameters [Out]"=w458:T29)  [unwired: 8 in]
        n145 = Unbundle By Name(w458) -> ("Manual Controls.Acquisition mode"=w460:T19, "Manual Controls.Save"=w459:bool)
        n146 = case shown="\"GPU FFT\"" w460 {
          tunnel: [w465 w473 w507 w540 w574 w608 w642 w676] -> w464
          tunnel: w461 -> [w465 w468 w502 w537 w571 w605 w639 w673]
          tunnel: w458 -> [_ w471 w505 w547 w581 w615 w649 w683]
          tunnel: w459 -> [_ w472 w506 w539 w573 w607 w641 w670]
          frame Default {
          }
          frame "GPU FFT" {
            n147 = call "FGV - Acquisition Status.vi"("Actions"=FGV_Actions."Get", "Error In"=w468) -> ("Error Out"=w467:errorcluster, "mem loc out"=w469:i32)  [unwired: 5 in, 3 out]
            n148 = case shown="2, Default" w469 {
              tunnel: [1 2] -> w466
              frame 2, Default {
              }
              frame 1 {
              }
            }
            n149 = case shown="2" w466 {
              tunnel: [w489 w494 w499] -> w479
              tunnel: w471 -> [_ w491 w497]
              tunnel: w472 -> [_ w490 w496]
              tunnel: w467 -> [w489 w493 w495]
              frame 0, Default {
              }
              frame 1 {
                # "memory block location"
                n150 = call "Save bline to memory1.vi"("action"=Save_Bline_to_Mem_Control."FFT and Save", "Save"=w490, "error in"=w493, "System Parameters"=w491) -> ("error out"=w494:errorcluster)  [unwired: 11 in]
              }
              frame 2 {
                # "memory block location"
                n151 = call "Save bline to memory2.vi"("action"=Save_Bline_to_Mem_Control."FFT and Save", "Save"=w496, "error in"=w495, "System Parameters"=w497) -> ("error out"=w499:errorcluster)  [unwired: 11 in]
              }
            }
            n152 = case shown="True" w472 {
              tunnel: w479 -> [w482 w484]
              tunnel: [w482 w483] -> w474
              frame False {
                # "do not save"
              }
              frame True {
                # "Save"
                n153 = Build Array(T26 {"Message"="Start", "Parameter"=variant} ("Message Packet Array")) -> (w486:T26[])
                n154 = call "Queue Manager.vi"("Queue Name"=QueueNames."Main Saving", "Action"=Queue_Manager_Actions."Enqueue", "Error In"=w484, "Message Packet Array"=w486) -> ("Error Out"=w483:errorcluster)  [unwired: 3 in, 4 out]
              }
            }
            n155 = Build Array(T26 {"Message"="Update Image", "Parameter"=variant} ("Message Packet Array")) -> (w476:T26[])
            n156 = call "Queue Manager.vi"("Queue Name"=QueueNames."Main Display", "Action"=Queue_Manager_Actions."Enqueue", "Error In"=w474, "Message Packet Array"=w476) -> ("Error Out"=w473:errorcluster)  [unwired: 3 in, 4 out]
          }
          frame "Alazar Spectral" {
            n157 = call "FGV - Acquisition Status.vi"("Actions"=FGV_Actions."Get", "Error In"=w502) -> ("Error Out"=w501:errorcluster, "mem loc out"=w503:i32)  [unwired: 5 in, 3 out]
            n158 = case shown="1" w503 {
              tunnel: [1 2] -> w500
              frame 2, Default {
              }
              frame 1 {
              }
            }
            n159 = case shown="2" w500 {
              tunnel: [w523 w528 w533] -> w513
              tunnel: w505 -> [_ w525 w531]
              tunnel: w506 -> [_ w524 w530]
              tunnel: w501 -> [w523 w527 w529]
              frame 0, Default {
              }
              frame 1 {
                # "memory block location"
                n160 = call "Save bline to memory1.vi"("action"=Save_Bline_to_Mem_Control."Alazar Spectral Save", "Save"=w524, "error in"=w527, "System Parameters"=w525) -> ("error out"=w528:errorcluster)  [unwired: 11 in]
              }
              frame 2 {
                # "memory block location"
                n161 = call "Save bline to memory2.vi"("action"=Save_Bline_to_Mem_Control."Alazar Spectral Save", "Save"=w530, "error in"=w529, "System Parameters"=w531) -> ("error out"=w533:errorcluster)  [unwired: 11 in]
              }
            }
            n162 = case shown="True" w506 {
              tunnel: w513 -> [w516 w518]
              tunnel: [w516 w517] -> w508
              frame False {
                # "do not save"
              }
              frame True {
                # "Save"
                n163 = Build Array(T26 {"Message"="Start", "Parameter"=variant} ("Message Packet Array")) -> (w520:T26[])
                n164 = call "Queue Manager.vi"("Queue Name"=QueueNames."Main Saving", "Action"=Queue_Manager_Actions."Enqueue", "Error In"=w518, "Message Packet Array"=w520) -> ("Error Out"=w517:errorcluster)  [unwired: 3 in, 4 out]
              }
            }
            n165 = Build Array(T26 {"Message"="Update Image", "Parameter"=variant} ("Message Packet Array")) -> (w510:T26[])
            n166 = call "Queue Manager.vi"("Queue Name"=QueueNames."Main Display", "Action"=Queue_Manager_Actions."Enqueue", "Error In"=w508, "Message Packet Array"=w510) -> ("Error Out"=w507:errorcluster)  [unwired: 3 in, 4 out]
          }
          frame "Alazar FFT" {
            n167 = call "FGV - Acquisition Status.vi"("Actions"=FGV_Actions."Get", "Error In"=w537) -> ("Error Out"=w536:errorcluster, "mem loc out"=w535:i32)  [unwired: 5 in, 3 out]
            n168 = case shown="1" w535 {
              tunnel: [1 2] -> w534
              frame 2, Default {
              }
              frame 1 {
              }
            }
            n169 = case shown="0, Default" w534 {
              tunnel: [w557 w562 w567] -> w546
              tunnel: w536 -> [w557 w561 w566]
              tunnel: w547 -> [_ w559 w564]
              tunnel: w539 -> [_ w558 w563]
              frame 0, Default {
              }
              frame 1 {
                # "memory block location"
                n170 = call "Save bline to memory1.vi"("action"=Save_Bline_to_Mem_Control."Save(PSOCT)", "Save"=w558, "error in"=w561, "System Parameters"=w559) -> ("error out"=w562:errorcluster)  [unwired: 11 in]
              }
              frame 2 {
                # "memory block location"
                n171 = call "Save bline to memory2.vi"("action"=Save_Bline_to_Mem_Control."Save(PSOCT)", "Save"=w563, "error in"=w566, "System Parameters"=w564) -> ("error out"=w567:errorcluster)  [unwired: 11 in]
              }
            }
            n172 = case shown="True" w539 {
              tunnel: w546 -> [w550 w552]
              tunnel: [w550 w551] -> w541
              frame False {
                # "do not save"
              }
              frame True {
                # "Save"
                n173 = Build Array(T26 {"Message"="Start", "Parameter"=variant} ("Message Packet Array")) -> (w554:T26[])
                n174 = call "Queue Manager.vi"("Queue Name"=QueueNames."Main Saving", "Action"=Queue_Manager_Actions."Enqueue", "Error In"=w552, "Message Packet Array"=w554) -> ("Error Out"=w551:errorcluster)  [unwired: 3 in, 4 out]
              }
            }
            n175 = Build Array(T26 {"Message"="Update Image", "Parameter"=variant} ("Message Packet Array")) -> (w543:T26[])
            n176 = call "Queue Manager.vi"("Queue Name"=QueueNames."Main Display", "Action"=Queue_Manager_Actions."Enqueue", "Error In"=w541, "Message Packet Array"=w543) -> ("Error Out"=w540:errorcluster)  [unwired: 3 in, 4 out]
          }
          frame "ThorOCT FFT" {
            n177 = call "FGV - Acquisition Status.vi"("Actions"=FGV_Actions."Get", "Error In"=w571) -> ("Error Out"=w570:errorcluster, "mem loc out"=w569:i32)  [unwired: 5 in, 3 out]
            n178 = case shown="1" w569 {
              tunnel: [1 2] -> w568
              frame 2, Default {
              }
              frame 1 {
              }
            }
            n179 = case shown="1" w568 {
              tunnel: [w591 w596 w601] -> w580
              tunnel: w570 -> [w591 w595 w600]
              tunnel: w581 -> [_ w593 w598]
              tunnel: w573 -> [_ w592 w597]
              frame 0, Default {
              }
              frame 1 {
                # "memory block location"
                n180 = call "Save bline to memory1.vi"("action"=Save_Bline_to_Mem_Control."Save(ThorOCT)", "Save"=w592, "error in"=w595, "System Parameters"=w593) -> ("error out"=w596:errorcluster)  [unwired: 11 in]
              }
              frame 2 {
                # "memory block location"
                n181 = call "Save bline to memory2.vi"("action"=Save_Bline_to_Mem_Control."Save(ThorOCT)", "Save"=w597, "error in"=w600, "System Parameters"=w598) -> ("error out"=w601:errorcluster)  [unwired: 11 in]
              }
            }
            n182 = case shown="True" w573 {
              tunnel: w580 -> [w584 w586]
              tunnel: [w584 w585] -> w575
              frame False {
                # "do not save"
              }
              frame True {
                # "Save"
                n183 = Build Array(T26 {"Message"="Start", "Parameter"=variant} ("Message Packet Array")) -> (w588:T26[])
                n184 = call "Queue Manager.vi"("Queue Name"=QueueNames."Main Saving", "Action"=Queue_Manager_Actions."Enqueue", "Error In"=w586, "Message Packet Array"=w588) -> ("Error Out"=w585:errorcluster)  [unwired: 3 in, 4 out]
              }
            }
            n185 = Build Array(T26 {"Message"="Update Image", "Parameter"=variant} ("Message Packet Array")) -> (w577:T26[])
            n186 = call "Queue Manager.vi"("Queue Name"=QueueNames."Main Display", "Action"=Queue_Manager_Actions."Enqueue", "Error In"=w575, "Message Packet Array"=w577) -> ("Error Out"=w574:errorcluster)  [unwired: 3 in, 4 out]
          }
          frame "ThorOCT Spectral" {
            n187 = call "FGV - Acquisition Status.vi"("Actions"=FGV_Actions."Get", "Error In"=w605) -> ("Error Out"=w604:errorcluster, "mem loc out"=w603:i32)  [unwired: 5 in, 3 out]
            n188 = case shown="1" w603 {
              tunnel: [1 2] -> w602
              frame 2, Default {
              }
              frame 1 {
              }
            }
            n189 = case shown="1" w602 {
              tunnel: [w625 w630 w635] -> w614
              tunnel: w604 -> [w625 w629 w634]
              tunnel: w615 -> [_ w627 w632]
              tunnel: w607 -> [_ w626 w631]
              frame 0, Default {
              }
              frame 1 {
                # "memory block location"
                n190 = call "Save bline to memory1.vi"("action"=Save_Bline_to_Mem_Control."ThorOCT Spectral Save", "Save"=w626, "error in"=w629, "System Parameters"=w627) -> ("error out"=w630:errorcluster)  [unwired: 11 in]
              }
              frame 2 {
                # "memory block location"
                n191 = call "Save bline to memory2.vi"("action"=Save_Bline_to_Mem_Control."ThorOCT Spectral Save", "Save"=w631, "error in"=w634, "System Parameters"=w632) -> ("error out"=w635:errorcluster)  [unwired: 11 in]
              }
            }
            n192 = case shown="True" w607 {
              tunnel: w614 -> [w618 w620]
              tunnel: [w618 w619] -> w609
              frame False {
                # "do not save"
              }
              frame True {
                # "Save"
                n193 = Build Array(T26 {"Message"="Start", "Parameter"=variant} ("Message Packet Array")) -> (w622:T26[])
                n194 = call "Queue Manager.vi"("Queue Name"=QueueNames."Main Saving", "Action"=Queue_Manager_Actions."Enqueue", "Error In"=w620, "Message Packet Array"=w622) -> ("Error Out"=w619:errorcluster)  [unwired: 3 in, 4 out]
              }
            }
            n195 = Build Array(T26 {"Message"="Update Image", "Parameter"=variant} ("Message Packet Array")) -> (w611:T26[])
            n196 = call "Queue Manager.vi"("Queue Name"=QueueNames."Main Display", "Action"=Queue_Manager_Actions."Enqueue", "Error In"=w609, "Message Packet Array"=w611) -> ("Error Out"=w608:errorcluster)  [unwired: 3 in, 4 out]
          }
          frame "ThorOCT B line" {
            n197 = call "FGV - Acquisition Status.vi"("Actions"=FGV_Actions."Get", "Error In"=w639) -> ("Error Out"=w638:errorcluster, "mem loc out"=w637:i32)  [unwired: 5 in, 3 out]
            n198 = case shown="1" w637 {
              tunnel: [1 2] -> w636
              frame 2, Default {
              }
              frame 1 {
              }
            }
            n199 = case shown="1" w636 {
              tunnel: [w659 w664 w669] -> w648
              tunnel: w638 -> [w659 w663 w668]
              tunnel: w649 -> [_ w661 w666]
              tunnel: w641 -> [_ w660 w665]
              frame 0, Default {
              }
              frame 1 {
                # "memory block location"
                n200 = call "Save bline to memory1.vi"("action"=Save_Bline_to_Mem_Control."Save(ThorOCT)", "Save"=w660, "error in"=w663, "System Parameters"=w661) -> ("error out"=w664:errorcluster)  [unwired: 11 in]
              }
              frame 2 {
                # "memory block location"
                n201 = call "Save bline to memory2.vi"("action"=Save_Bline_to_Mem_Control."Save(ThorOCT)", "Save"=w665, "error in"=w668, "System Parameters"=w666) -> ("error out"=w669:errorcluster)  [unwired: 11 in]
              }
            }
            n202 = case shown="True" w641 {
              tunnel: w648 -> [w652 w654]
              tunnel: [w652 w653] -> w643
              frame False {
                # "do not save"
              }
              frame True {
                # "Save"
                n203 = Build Array(T26 {"Message"="Start", "Parameter"=variant} ("Message Packet Array")) -> (w656:T26[])
                n204 = call "Queue Manager.vi"("Queue Name"=QueueNames."Main Saving", "Action"=Queue_Manager_Actions."Enqueue", "Error In"=w654, "Message Packet Array"=w656) -> ("Error Out"=w653:errorcluster)  [unwired: 3 in, 4 out]
              }
            }
            n205 = Build Array(T26 {"Message"="Update Image", "Parameter"=variant} ("Message Packet Array")) -> (w645:T26[])
            n206 = call "Queue Manager.vi"("Queue Name"=QueueNames."Main Display", "Action"=Queue_Manager_Actions."Enqueue", "Error In"=w643, "Message Packet Array"=w645) -> ("Error Out"=w642:errorcluster)  [unwired: 3 in, 4 out]
          }
          frame "Alazar B line" {
            n207 = call "FGV - Acquisition Status.vi"("Actions"=FGV_Actions."Get", "Error In"=w673) -> ("Error Out"=w672:errorcluster, "mem loc out"=w674:i32)  [unwired: 5 in, 3 out]
            n208 = case shown="2, Default" w674 {
              tunnel: [1 2] -> w671
              frame 2, Default {
              }
              frame 1 {
              }
            }
            n209 = case shown="1" w671 {
              tunnel: [w693 w698 w703] -> w682
              tunnel: w672 -> [w693 w697 w702]
              tunnel: w683 -> [_ w695 w700]
              tunnel: w670 -> [_ w694 w699]
              frame 0, Default {
              }
              frame 1 {
                # "memory block location"
                n210 = call "Save bline to memory1.vi"("action"=Save_Bline_to_Mem_Control."Save(PSOCT)", "Save"=w694, "error in"=w697, "System Parameters"=w695) -> ("error out"=w698:errorcluster)  [unwired: 11 in]
              }
              frame 2 {
                # "memory block location"
                n211 = call "Save bline to memory2.vi"("action"=Save_Bline_to_Mem_Control."Save(PSOCT)", "Save"=w699, "error in"=w702, "System Parameters"=w700) -> ("error out"=w703:errorcluster)  [unwired: 11 in]
              }
            }
            n212 = case shown="False" w670 {
              tunnel: w682 -> [w686 w688]
              tunnel: [w686 w687] -> w677
              frame False {
                # "do not save"
              }
              frame True {
                # "Save"
                n213 = Build Array(T26 {"Message"="Start", "Parameter"=variant} ("Message Packet Array")) -> (w690:T26[])
                n214 = call "Queue Manager.vi"("Queue Name"=QueueNames."Main Saving", "Action"=Queue_Manager_Actions."Enqueue", "Error In"=w688, "Message Packet Array"=w690) -> ("Error Out"=w687:errorcluster)  [unwired: 3 in, 4 out]
              }
            }
            n215 = Build Array(T26 {"Message"="Update Image", "Parameter"=variant} ("Message Packet Array")) -> (w679:T26[])
            n216 = call "Queue Manager.vi"("Queue Name"=QueueNames."Main Display", "Action"=Queue_Manager_Actions."Enqueue", "Error In"=w677, "Message Packet Array"=w679) -> ("Error Out"=w676:errorcluster)  [unwired: 3 in, 4 out]
          }
        }
      }
    }
    n217 = call "Error Message Handler.vi"("Error In"=w446) -> ("Error Out"=w450:errorcluster, "T button?"=w448:bool)  [unwired: 9 in]
    n218 = case shown="False" w448 {
      tunnel: w450 -> [w704 w706]
      tunnel: [w704 w707] -> w449
      frame False {
      }
      frame True {
        n219 = call "Queue Manager.vi"("Queue Name"=QueueNames."Main Processing", "Action"=Queue_Manager_Actions."Enqueue", "Error In"=w706, "Message Packet Array"=T26[] [{"Message"="Exit", "Parameter"=variant}] ("Message Packet [In]")) -> ("Error Out"=w707:errorcluster)  [unwired: 3 in, 4 out]
      }
    }
  }
  n220 = while {
    shift-right: [w711] -> w18
    shift-left: w4 -> [w720]
    stop <- w721 stop-if-true
    # "Main GUI"
    n221 = call "Queue Manager.vi"("Queue Name"=QueueNames."Main GUI", "Action"=Queue_Manager_Actions."Dequeue", "Error In"=w720) -> ("Error Out"=w718:errorcluster, "Message Packet [Out]"=w717:T26)  [unwired: 4 in, 3 out]
    n222 = Unbundle(w717) -> ("Message"=w714:string, "Parameter"=w716:variant)
    n223 = case shown="\"Wait for User Input\"" w714 {
      tunnel: w718 -> [w736 w768 w779 w806 w825 w839 w852 w970 w978]
      tunnel: w716 -> [_ _ _ _ _ _ _ _ _]
      tunnel: [w735 w764 w775 w798 w821 w837 w853 w968 w978] -> w710
      tunnel: [_ _ _ _ _ _ _ TRUE _] -> w721
      frame "Init" {
        n224 = call "Queue Manager.vi"("Queue Name"=QueueNames."Main GUI", "Action"=Queue_Manager_Actions."Enqueue", "Error In"=w736, "Message Packet Array"=T26[] [{"Message"="Init Variables", "Parameter"=variant}, {"Message"="Set Front Panel", "Parameter"=variant}, {"Message"="Update User Settings", "Parameter"=variant}, {"Message"="Configure Hardware", "Parameter"=variant}, {"Message"="Wait for Complete", "Parameter"=variant}, {"Message"="Wait for User Input", "Parameter"=variant}]) -> ("Error Out"=w735:errorcluster)  [unwired: 3 in, 4 out]
      }
      frame "Init Variables" {
        n225 = call "Status Queue.vi"("Action"=Queue_Manager_Actions."Enqueue", "Error In"=w768, "Status Message [In]"="Initializing Variables...") -> ("Error Out"=w763:errorcluster)  [unwired: 7 in, 1 out]
        n226 = control-ref of="This VI"() -> (w766:refnum<vi>)
        n227 = call "Defer Panel Updates.vi"("Action"=enum16{"Init", "Freeze", "Unfreeze"}."Init", "Error In"=w763, "reference"=w766) -> ("Error Out"=w753:errorcluster)  [unwired: 8 in]
        n228 = call "Image Queue.vi"("Action"=Queue_Manager_Actions."Init", "Error In"=w753) -> ("Error Out"=w752:errorcluster)  [unwired: 8 in, 1 out]
        n229 = call "System Parameters - FGV.vi"("Actions"=FGV_Actions."Init", "Error In"=w752) -> ("Error Out"=w748:errorcluster)  [unwired: 8 in, 1 out]
        n230 = call "Tile naming.vi"(7:Tile_naming_actions."Init", "Error In"=w748) -> ("Error Out"=w746:errorcluster)  [unwired: 7 in, 2 out]
        n231 = call "Display Data Queue.vi"("max queue size (-1, unlimited)"=3, "Action"=Queue_Manager_Actions."Init", "error in (no error)"=w746) -> ("error out"=w741:errorcluster)  [unwired: 5 in, 3 out]
        n232 = call "Error output.vi"("Actions"=FGV_Actions."Init") -> ()  [unwired: 8 in, 3 out]
        n233 = call "Spectral Save Queue.vi"("max queue size (-1, unlimited)"=3, "Action"=Queue_Manager_Actions."Init", "error in (no error)"=w741) -> ("error out"=w740:errorcluster)  [unwired: 5 in, 3 out]
        n234 = call "Save Data Queue.vi"("max queue size (-1, unlimited)"=3, "Action"=Queue_Manager_Actions."Init", "error in (no error)"=w740) -> ("error out"=w751:errorcluster)  [unwired: 5 in, 3 out]
        n235 = call "Process status.vi"("Actions"=FGV_Actions."Init") -> ()  [unwired: 9 in, 2 out]
        n236 = disable-structure shown="Enabled" {
          disable-tunnel: [w771 w774] -> w743
          disable-tunnel: w751 -> [w770 w774]
          frame Enabled {
            n237 = call "Read Config from File.vi"("error in (no error)"=w770) -> ("error out"=w773:errorcluster, "System Parameters"=w769:T29)  [unwired: 9 in]
            n238 = call "System Parameters - FGV.vi"("Actions"=FGV_Actions."Set", "Error In"=w773, "System Parameters [In]"=w769) -> ("Error Out"=w771:errorcluster)  [unwired: 7 in, 1 out]
          }
          frame Disabled {
          }
        }
        n239 = control-ref of="Imaging Parameter"() -> (w756:refnum<vi>)
        n240 = call "Set Front Panel Custom Image Size Cluster Control.vi"("error in (no error)"=w743, "Enable/Disable"=FALSE, "Init"=TRUE, "Cluster Ref In"=w756) -> ("error IO"=w758:errorcluster)  [unwired: 7 in]
        n241 = call "FGV - Acquisition Status.vi"("Actions"=FGV_Actions."Init", "Error In"=w758) -> ("Error Out"=w764:errorcluster, "Scan Type [Out]"=w759:T6)  [unwired: 5 in, 3 out]
        n242 = local write "Scan Type"(w759) -> ()
      }
      frame "Set Front Panel" {
        n243 = call "Status Queue.vi"("Action"=Queue_Manager_Actions."Enqueue", "Error In"=w779, "Status Message [In]"="Setting Front Panel Controls...") -> ("Error Out"=w780:errorcluster)  [unwired: 7 in, 1 out]
        n244 = call "Defer Panel Updates.vi"("Action"=enum16{"Init", "Freeze", "Unfreeze"}."Freeze", "Error In"=w780) -> ("Error Out"=w788:errorcluster)  [unwired: 9 in]
        n245 = call "FGV - Acquisition Status.vi"("Actions"=FGV_Actions."Get", "Error In"=w788) -> ("Error Out"=w785:errorcluster, "Scan Type [Out]"=w783:T6, "Level Status out"=w784:bool)  [unwired: 5 in, 2 out]
        n246 = case "Acquiring?" shown="True" w784 {
          tunnel: [w792 w797] -> w786
          tunnel: w785 -> [w793 w797]
          tunnel: w783 -> [w791 _]
          frame False {
            # "Non-Acquiring FP States"
            n247 = disable-structure shown="Enabled" {
              disable-tunnel: w793 -> [w796 _]
              disable-tunnel: [w795 _] -> w792
              disable-tunnel: w791 -> [w794 _]
              frame Disabled {
                n248 = call "Set Main GUI for Different Acquire States.vi"("Error In"=w796, "Scan Type [Out]"=w794) -> ("Error Out"=w795:errorcluster)  [unwired: 9 in]
              }
              frame Enabled {
              }
            }
          }
          frame True {
            # "Acquiring FP States"
          }
        }
        n249 = call "Defer Panel Updates.vi"("Action"=enum16{"Init", "Freeze", "Unfreeze"}."Unfreeze", "Error In"=w786) -> ("Error Out"=w776:errorcluster)  [unwired: 9 in]
        n250 = call "Status Queue.vi"("Action"=Queue_Manager_Actions."Enqueue", "Error In"=w776, "Status Message [In]"="Finished Setting Front Panel.") -> ("Error Out"=w775:errorcluster)  [unwired: 7 in, 1 out]
      }
      frame "Update User Settings" {
        n251 = disable-structure shown="Enabled" {
          disable-tunnel: [Queue_Manager_Actions."Enqueue" ("Action") Queue_Manager_Actions."Enqueue" ("Action")] -> w800
          frame Enabled {
            n252 = call "System Parameters - FGV.vi"("Actions"=FGV_Actions."Get") -> ("System Parameters [Out]"=w818:T29)  [unwired: 9 in, 1 out]
            n253 = Unbundle By Name(w818) -> ("Optical Parameters"=w816:T2, "Vibratome"=w815:T15, "Table Stages"=w814:T20, "Imaging Parameter"=w813:T4, "Galvo HW Parameters"=w812:T3, "Alazar parameters"=w811:T7, "Mosaic Paramter"=w810:T33, "Vibratome Axis"=w809:T14, "Manual Controls"=w808:T17)
            n254 = local write "Galvo HW Parameters"(w812) -> ()
            n255 = local write "Alazar parameters"(w811) -> ()
            n256 = local write "Imaging Parameter"(w813) -> ()
            n257 = local write "Optical Parameters"(w816) -> ()
            n258 = local write "Manual Controls"(w808) -> ()
            n259 = local write "Mosaic Paramter"(w810) -> ()
            n260 = local write "Vibratome"(w815) -> ()
            n261 = local write "Vibratome Axis"(w809) -> ()
            n262 = local write "Table Stages"(w814) -> ()
          }
          frame Disabled {
          }
        }
        n263 = call "Status Queue.vi"("Action"=w800, "Error In"=w806, "Status Message [In]"="Loading User Settings...") -> ("Error Out"=w804:errorcluster)  [unwired: 7 in, 1 out]
        n264 = call "Defer Panel Updates.vi"("Action"=enum16{"Init", "Freeze", "Unfreeze"}."Freeze", "Error In"=w804) -> ("Error Out"=w799:errorcluster)  [unwired: 9 in]
        n265 = call "Set Front Panel Custom Image Size Cluster Control.vi"("error in (no error)"=w799, "Enable/Disable"=TRUE) -> ("error IO"=w802:errorcluster)  [unwired: 9 in]
        n266 = call "Defer Panel Updates.vi"("Action"=enum16{"Init", "Freeze", "Unfreeze"}."Unfreeze", "Error In"=w802) -> ("Error Out"=w798:errorcluster)  [unwired: 9 in]
      }
      frame "Configure Hardware" {
        n267 = call "Status Queue.vi"("Action"=Queue_Manager_Actions."Enqueue", "Error In"=w825, "Status Message [In]"="Initializing Hardware...") -> ("Error Out"=w824:errorcluster)  [unwired: 7 in, 1 out]
        n268 = Build Array(T26 {"Message"="Init Hardware", "Parameter"=variant} ("Message Packet [In]")) -> (w822:T26[])
        n269 = call "Queue Manager.vi"("Queue Name"=QueueNames."Main Scan Processor", "Action"=Queue_Manager_Actions."Enqueue", "Error In"=w824, "Message Packet Array"=w822) -> ("Error Out"=w821:errorcluster)  [unwired: 3 in, 4 out]
      }
      frame "Wait for Complete" {
        n270 = call "TickTock.vi"("Error In"=w839) -> ("Error Out"=w835:errorcluster, "Current Time (Out)"=w834:timestamp)  [unwired: 8 in, 1 out]
        n271 = while {
          shift-right: [w842] -> w836
          shift-left: w835 -> [w850]
          tunnel: w834 -> [w849]
          tunnel: [w840] -> w833
          stop <- w841 stop-if-true
          n272 = call "Inline Wait.vi"("Error In"=w850, "milliseconds to wait"=u32 100) -> ("Error Out"=w846:errorcluster)  [unwired: 9 in]
          n273 = call "TickTock.vi"("Error In"=w846, "Current Time (In)"=w849) -> ("Error Out"=w842:errorcluster, "dt"=w848:dbl)  [unwired: 7 in, 1 out]
          n274 = Greater?(x=60000.0, y=w848) -> (0:w840:bool)
          n275 = global read "Main Scan Processor Status.vi" "Busy"() -> (w844:bool)
          n276 = Not(x=w844) -> (.not. x?=w843:bool)
          n277 = Or(x=w840, y=w843) -> (x .or. y?=w841:bool)
        }
        n278 = Select(t="Completed." ("Status Message [In]"), s=w833, f="Operation timed out." ("Status Message [In]")) -> (s? t:f=w830:string)
        n279 = call "Status Queue.vi"("Action"=Queue_Manager_Actions."Enqueue", "Error In"=w836, "Status Message [In]"=w830) -> ("Error Out"=w837:errorcluster)  [unwired: 7 in, 1 out]
      }
      frame "Wait for User Input" {
        n280 = event shown="[0] Timeout" {
          selector: _ -> [_ _ _ _ _ _]
          dyn-events: _ -> [_ _ _ _ _ _]
          timeout: 100 -> [_ _ _ _ _ _]
          tunnel: [w862 w899 w909 w925 w939 w956] -> w853
          tunnel: w852 -> [w867 w888 w911 w922 w943 w957]
          event Timeout {
            n281 = event-data() -> ()  [unwired: 1 in, 3 out]
            n282 = Unbundle By Name("Imaging Parameter") -> ("Custom Size.X"=w855:u16, "Custom Size.Y"=w858:u16)
            n283 = To Unsigned Quad Integer(1:w858) -> (0:w857:u64)
            n284 = To Unsigned Quad Integer(1:w855) -> (0:w856:u64)
            n285 = Add(x=w856, y=u16 50) -> (x+y=w854:u64)
            n286 = Multiply(x=w854, y=w857) -> (x*y=w860:u64)
            n287 = Bundle By Name(cluster="Alazar parameters", "Acq Settings.Records Per Buffer"=w854, "Acq Settings.Records Count (Records/Acq)"=w860) -> (w875:T7)
            n288 = call "System Parameters - FGV.vi"("Actions"=FGV_Actions."Get", "Error In"=w867) -> ("Error Out"=w872:errorcluster, "System Parameters [Out]"=w871:T29)  [unwired: 8 in]
            n289 = Bundle By Name(cluster=w871, "Vibratome"="Vibratome", "Optical Parameters"="Optical Parameters", "Imaging Parameter"="Imaging Parameter", "Galvo HW Parameters"="Galvo HW Parameters", "Alazar parameters"=w875, "Table Stages"="Table Stages", "Mosaic Paramter"="Mosaic Paramter", "Vibratome Axis"="Vibratome Axis", "Manual Controls"="Manual Controls") -> (w874:T29)
            n290 = call "System Parameters - FGV.vi"("Actions"=FGV_Actions."Set", "Error In"=w872, "System Parameters [In]"=w874) -> ("Error Out"=w863:errorcluster)  [unwired: 7 in, 1 out]
            n291 = call "Queue Manager.vi"("Queue Name"=QueueNames."Main GUI", "Action"=Queue_Manager_Actions."Enqueue", "Error In"=w863, "Message Packet Array"=T26[] [{"Message"="Wait for User Input", "Parameter"=variant}]) -> ("Error Out"=w862:errorcluster)  [unwired: 3 in, 4 out]
          }
          event "Quit": Value Change {
            n292 = event-data() -> ()  [unwired: 1 in, 1 out]
            n293 = call "FGV - Acquisition Status.vi"("Actions"=FGV_Actions."Get", "Error In"=w888) -> ("Error Out"=w887:errorcluster, "Scan Type [Out]"=w885:T6, "mem loc out"=w882:i32)  [unwired: 5 in, 2 out]
            n294 = call "FGV - Acquisition Status.vi"("mem loc"=w882, "Actions"=FGV_Actions."Set", "Error In"=w887, "Quit status"=TRUE, "Scan Type [In]"=w885, "Level Status In"=FALSE ("Status In")) -> ("Error Out"=w886:errorcluster)  [unwired: 1 in, 4 out]
            n295 = call "Queue Manager.vi"("Action"=Queue_Manager_Actions."Flush All Queues", "Error In"=w886) -> ("Error Out"=w891:errorcluster)  [unwired: 5 in, 4 out]
            n296 = call "Status Queue.vi"("Action"=Queue_Manager_Actions."Enqueue", "Error In"=w891, "Status Message [In]"="Exiting Software...") -> ("Error Out"=w895:errorcluster)  [unwired: 7 in, 1 out]
            n297 = disable-structure shown="Disabled" {
              disable-tunnel: w895 -> [w902 w903]
              disable-tunnel: [w901 w903] -> w894
              frame Disabled {
                n298 = call "Set Main GUI for Different Acquire States.vi"("Error In"=w902, "Scan Type [Out]"=ScanType."Single Frame") -> ("Error Out"=w901:errorcluster)  [unwired: 9 in]
              }
              frame Enabled {
              }
            }
            n299 = call "Queue Manager.vi"("Action"=Queue_Manager_Actions."Enqueue All", "Error In"=w894, "Message Packet Array"=T26[] [{"Message"="Exit", "Parameter"=variant}] ("Message Packet [In]")) -> ("Error Out"=w899:errorcluster)  [unwired: 4 in, 4 out]
          }
          event "AIP": Value Change {
            w912 = 2 items=["No Event"=0, "Click Event"=1, "Draw Event"=2, "Size Event"=4, "Scroll Event"=5, "Double Click Event"=8]
            n300 = event-data() -> ("CtlRef"=w904:refnum<vi>)  [unwired: 1 in, 5 out]
            n301 = Build Array(w912) -> (w913:i32[])
            n302 = invoke class="ImageControl" method="Get Last Event"(reference=w904, error in=w911, "Which Events"=w913) -> (error out=w910:errorcluster)  [unwired: 5 in, 7 out]
            n303 = Build Array(T26 {"Message"="Wait for User Input", "Parameter"=variant} ("Message Packet [In]")) -> (w905:T26[])
            n304 = call "Queue Manager.vi"("Queue Name"=QueueNames."Main GUI", "Action"=Queue_Manager_Actions."Enqueue", "Error In"=w910, "Message Packet Array"=w905) -> ("Error Out"=w909:errorcluster)  [unwired: 3 in, 4 out]
          }
          event Value Change {
            n305 = event-data() -> ("NewVal"=w918:T34)  [unwired: 1 in]
            n306 = Add(x=w918, y=5) -> (x+y=w931:i32)
            n307 = call "System Parameters - FGV.vi"("Actions"=FGV_Actions."Get", "Error In"=w922) -> ("Error Out"=w921:errorcluster, "System Parameters [Out]"=w919:T29)  [unwired: 8 in]
            n308 = Power Of 2(x=w931) -> (2^x=w930:dbl)
            n309 = Bundle By Name(cluster=w919, "Imaging Parameter.XY Image Size"=w918) -> (w914:T29)
            n310 = local read "Imaging Parameter"() -> (w917:T4)
            n311 = To Unsigned Word Integer(number=w930) -> (unsigned 16bit integer=w915:u16)
            n312 = Bundle By Name(cluster=w917, "Custom Size.X"=w915, "Custom Size.Y"=w915) -> (w916:T4)
            n313 = local write "Imaging Parameter"(w916) -> ()
            n314 = call "System Parameters - FGV.vi"("Actions"=FGV_Actions."Set", "Error In"=w921, "System Parameters [In]"=w914) -> ("Error Out"=w920:errorcluster)  [unwired: 7 in, 1 out]
            n315 = Build Array(T26 {"Message"="Wait for User Input", "Parameter"=variant} ("Message Packet [In]")) -> (w926:T26[])
            n316 = call "Queue Manager.vi"("Queue Name"=QueueNames."Main GUI", "Action"=Queue_Manager_Actions."Enqueue", "Error In"=w920, "Message Packet Array"=w926) -> ("Error Out"=w925:errorcluster)  [unwired: 3 in, 4 out]
          }
          event Value Change {
            n317 = event-data() -> ()  [unwired: 1 in, 6 out]
            n318 = call "FGV - Acquisition Status.vi"("Actions"=FGV_Actions."Get") -> ("Level Status out"=w938:bool, "mem loc out"=w933:i32)  [unwired: 6 in, 3 out]
            n319 = call "FGV - Acquisition Status.vi"("mem loc"=w933, "Actions"=FGV_Actions."Set", "Quit status"=FALSE, "Scan Type [In]"="Scan Type", "Level Status In"=w938) -> ()  [unwired: 2 in, 5 out]
            n320 = call "Queue Manager.vi"("Queue Name"=QueueNames."Main GUI", "Action"=Queue_Manager_Actions."Enqueue", "Error In"=w943, "Message Packet Array"=T26[] [{"Message"="Set Front Panel", "Parameter"=variant}, {"Message"="Wait for User Input", "Parameter"=variant}]) -> ("Error Out"=w939:errorcluster)  [unwired: 3 in, 4 out]
          }
          event "Acquire": Value Change {
            n321 = event-data() -> ()  [unwired: 1 in, 6 out]
            n322 = call "Queue Manager.vi"("Queue Name"=QueueNames."Main GUI", "Action"=Queue_Manager_Actions."Enqueue", "Error In"=w957, "Message Packet Array"=T26[] [{"Message"="Wait for User Input", "Parameter"=variant}]) -> ("Error Out"=w946:errorcluster)  [unwired: 3 in, 4 out]
            n323 = call "FGV - Acquisition Status.vi"("Actions"=FGV_Actions."Get", "Error In"=w946) -> ("Error Out"=w947:errorcluster, "Scan Type [Out]"=w948:T6, "Level Status out"=w949:bool, "mem loc out"=w944:i32)  [unwired: 5 in, 1 out]
            n324 = Not(x=w949) -> (.not. x?=w950:bool)
            n325 = call "FGV - Acquisition Status.vi"("mem loc"=w944, "Actions"=FGV_Actions."Set", "Error In"=w947, "Quit status"=FALSE, "Scan Type [In]"=w948, "Level Status In"=w950) -> ()  [unwired: 1 in, 5 out]
            n326 = case "Start Acquisition?" shown="False" w949 {
              tunnel: w946 -> [w958 w966]
              tunnel: [w959 w966] -> w956
              frame False {
                # "Starts Acquisition if Current Acquisition Status is \"Off\""
                n327 = call "Queue Manager.vi"("Queue Name"=QueueNames."Main Scan Processor", "Action"=Queue_Manager_Actions."Enqueue", "Error In"=w958, "Message Packet Array"=T26[] [{"Message"="Acquire", "Parameter"=variant}] ("Message Packet [In]")) -> ("Error Out"=w960:errorcluster)  [unwired: 3 in, 4 out]
                n328 = call "Status Queue.vi"("Action"=Queue_Manager_Actions."Enqueue", "Error In"=w960, "Status Message [In]"="Scanning...") -> ("Error Out"=w959:errorcluster)  [unwired: 7 in, 1 out]
              }
              frame True {
                # "Stops Acquisition if Current Status is On"
              }
            }
          }
        }
      }
      frame "Exit" {
        n329 = disable-structure shown="Enabled" {
          disable-tunnel: w970 -> [w976 w977]
          disable-tunnel: [w973 w977] -> w967
          frame Enabled {
            n330 = call "System Parameters - FGV.vi"("Actions"=FGV_Actions."Get", "Error In"=w976) -> ("Error Out"=w975:errorcluster, "System Parameters [Out]"=w972:T29)  [unwired: 8 in]
            n331 = call "Write Config to File.vi"("error in (no error)"=w975, "System Parameters"=w972) -> ("error out"=w973:errorcluster)  [unwired: 9 in]
          }
          frame Disabled {
          }
        }
        n332 = call "Save Data Queue.vi"("Action"=Queue_Manager_Actions."Release Queue", "error in (no error)"=w967) -> ("error out"=w968:errorcluster)  [unwired: 6 in, 3 out]
      }
      frame Default {
      }
    }
    n333 = call "Error Message Handler.vi"("Error In"=w710) -> ("Error Out"=w713:errorcluster, "T button?"=w712:bool)  [unwired: 9 in]
    n334 = case shown="False" w712 {
      tunnel: w713 -> [w722 w723]
      tunnel: [w722 w724] -> w711
      frame False {
      }
      frame True {
        n335 = call "Status Queue.vi"("Action"=Queue_Manager_Actions."Enqueue", "Error In"=w723, "Status Message [In]"="Exiting Software...") -> ("Error Out"=w728:errorcluster)  [unwired: 7 in, 1 out]
        n336 = call "Set Main GUI for Different Acquire States.vi"("Error In"=w728, "Scan Type [Out]"=ScanType."Single Frame") -> ("Error Out"=w727:errorcluster)  [unwired: 9 in]
        n337 = call "Queue Manager.vi"("Action"=Queue_Manager_Actions."Enqueue All", "Error In"=w727, "Message Packet Array"=T26[] [{"Message"="Exit", "Parameter"=variant}] ("Message Packet [In]")) -> ("Error Out"=w724:errorcluster)  [unwired: 4 in, 4 out]
      }
    }
  }
  n338 = call "Queue Manager.vi"("Queue Name"=QueueNames."Main Display", "Action"=Queue_Manager_Actions."Release Queue", "Error In"=w11) -> ()  [unwired: 4 in, 5 out]
  n339 = call "Queue Manager.vi"("Queue Name"=QueueNames."Main Processing", "Action"=Queue_Manager_Actions."Release Queue", "Error In"=w5) -> ()  [unwired: 4 in, 5 out]
  n340 = call "Queue Manager.vi"("Queue Name"=QueueNames."Main Saving", "Action"=Queue_Manager_Actions."Release Queue", "Error In"=w7) -> ()  [unwired: 4 in, 5 out]
  n341 = call "Queue Manager.vi"("Queue Name"=QueueNames."Main Scan Processor", "Action"=Queue_Manager_Actions."Release Queue", "Error In"=w13) -> ()  [unwired: 4 in, 5 out]
  n342 = call "Queue Manager.vi"("Queue Name"=QueueNames."Main GUI", "Action"=Queue_Manager_Actions."Release Queue", "Error In"=w18) -> ()  [unwired: 4 in, 5 out]
